vi "resonant.calculation vi_rrMD.vi"() -> ()   [LabVIEW 2012]
doc: "SciScan 1.2 160622"
uses:
  CommonResource VIs/Timing/Timer Commands.ctl
  Custom Controls/display palette control.ctl
  Custom Controls/scan mode main settings tab.ctl
  Custom Controls/pixel resolution resonant enum.ctl
  Custom Controls/MAIN Image panel reso tab Control type def.ctl
  Custom Controls/experiment type.ctl
  Custom Controls/advanced settings inner tab CTL.ctl
  Plugins/Macro Module/Macro Rule/subVIs/MacroRules_FGV_Commands.ctl
  Custom Controls/Histogram tab reso.ctl
  <vilib>/Utility/VariantDataType/Type.ctl
  GFG/GFGstringGet.vi
  GFG/GFGfpRefGet.vi
  GFG/GFGbooleanGet.vi
  GFG/GFGnumericGet.vi
  GFG/GFGDisplayRefsGet.vi
  GFG/GFGImageRefsGet.vi
  GFG/GFG library.lvlib
  <vilib>/Utility/VariantDataType/VariantType.lvlib
panel:
  out "Source VI 2":string
  out "ready for flystart?":bool
  out "Iteration":i32
  in  "String":string
  out "Source VI":string
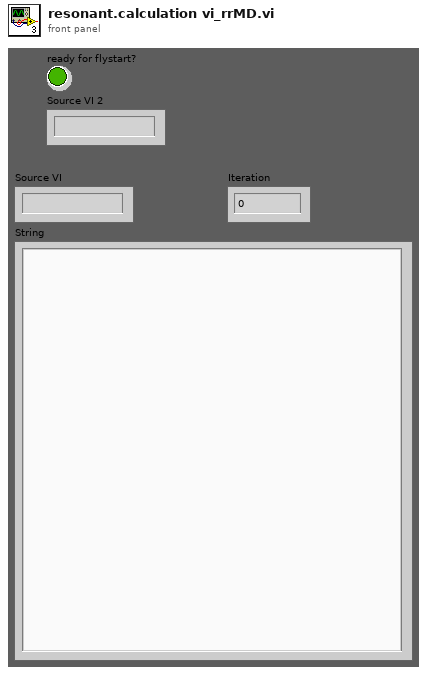
[diagram p1: front panel]
types:
  T1 = typedef "Timer Commands.ctl" = enum16{"Clear All", "Start", "Pause", "Check Time"}
  T2 = cluster{"WaveformChartRef":refnum<vi>, "DigitalRef":refnum<vi>, "ArrayRef":refnum<vi>, "TabControlRef":refnum<vi>, "EnumRef":refnum<vi>, "RingRef":refnum<vi>, "BooleanRef":refnum<vi>, "KnobRef":refnum<vi>, "SlideRef":refnum<vi>, "PathRef":refnum<vi>, "StringRef":refnum<vi>, "ComboBox":refnum<vi>, "WaveformGraphRef":refnum<vi>}
  T3 = typedef "display palette control.ctl" = enum16{"standard", "high clipping red", "low clipping blue", "high and low clipping", "high / low (full range)"}
  T4 = typedef "scan mode main settings tab.ctl" = enum32{"2D frame", "2D line scan", "general settings", "Z Stack", "piezo"}
  T5 = enum8{"Enabled", "Disabled", "Disabled and Grayed Out"}
  T6 = typedef "MAIN Image panel reso tab Control type def.ctl" = enum32{"Channel 1", "Channel 2", "Channel 3", "Channel 4", "Channel 5", "all channels", "RGB overlay", "ROI", "arbitrary line scan"}
  T7 = typedef "experiment type.ctl" = string
  T8 = enum32{"Page Enabled", "Page Disabled", "Page Disabled & Grayed"}
  T9 = typedef "advanced settings inner tab CTL.ctl" = enum32{"arb. frames", "AO", "AI", "channels", "trigger", "Zstack data"}
  T10 = typedef "MacroRules_FGV_Commands.ctl" = enum16{"Read File", "Get All", "Get Param and Flags"}
  T11 = typedef "Histogram tab reso.ctl" = enum32{"hist Ch 1", "hist Ch 4", "hist Ch 5", "hist Ch 3", "hist Ch 2"}
  T12 = cluster{"Channel 1 small":refnum<vi>, "Channel 2 small":refnum<vi>, "Channel 3 small":refnum<vi>, "Channel 4 small":refnum<vi>, "Channel 1 large":refnum<vi>, "Channel 2 large":refnum<vi>, "Channel 3 large":refnum<vi>, "Channel 4 large":refnum<vi>, "RGB overlay":refnum<vi>, "ROI Image display":refnum<vi>, "arb line scan display":refnum<vi>, "Channel 5 large":refnum<vi>}
  T13 = typedef "pixel resolution resonant enum.ctl" = enum16{"512 x  64", "512 x 128", "512 x 256", "512 x 512", "512 x arbitrary", "1024 x 512", "1024 x 1024", " 1024 x arbitrary", " 1536 x  512", " 1536 x arbitrary"}
  T14 = typedef "biotfile select.ctl" = enum16{"7962with5751_512px_40Mhz", "7962with5751_512px_50Mhz", "7961with5734_1024px_120Mhz or ext lasersync", "7962with5734_1024px_120Mhz or ext lasersync", "7962with5734_512px_120Mhz or ext lasersync", "7961with5734_512px_120Mhz or ext lasersync", "7962with5751_12kHz_512px_50MHz_4ch", "7962with5751_1536px_2ch_40Mhz", "7962with5751_1536px_2ch_50Mhz", "7962with5751_12kHz_1024px_2ch_50MHz"}
  T15 = typedef "LVStringsAndValuesArrayTypeDef.ctl" = cluster{"String":string, "Value":ext}[]
  T16 = typedef "IMAQ Image.ctl" = refnum<image>
  T17 = cluster{"Channel 1 small":T16, "Channel 2 small":T16, "Channel 3 small":T16, "Channel 4 small":T16, "Channel 1 large":T16, "Channel 2 large":T16, "Channel 3 large":T16, "Channel 4 large":T16, "RGB overlay":T16, "ROI Image display":T16, "arb line scan display":T16, "Channel 5 large":T16}
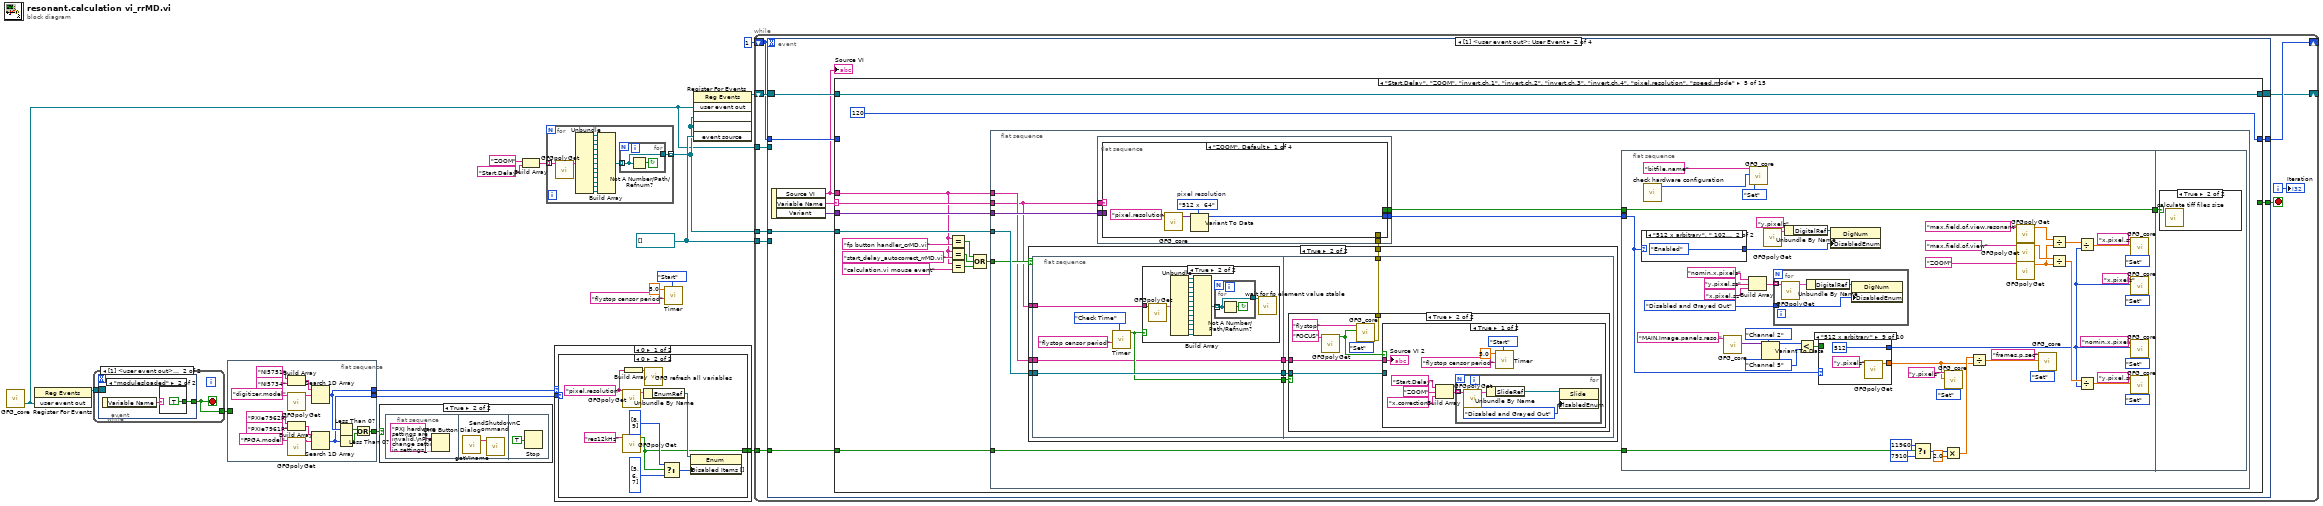
[diagram p0: block diagram]
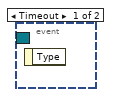
[diagram p3: hidden frame]
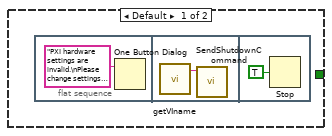
[diagram p5: hidden frame]
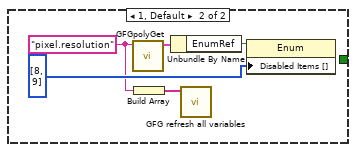
[diagram p6: hidden frame]
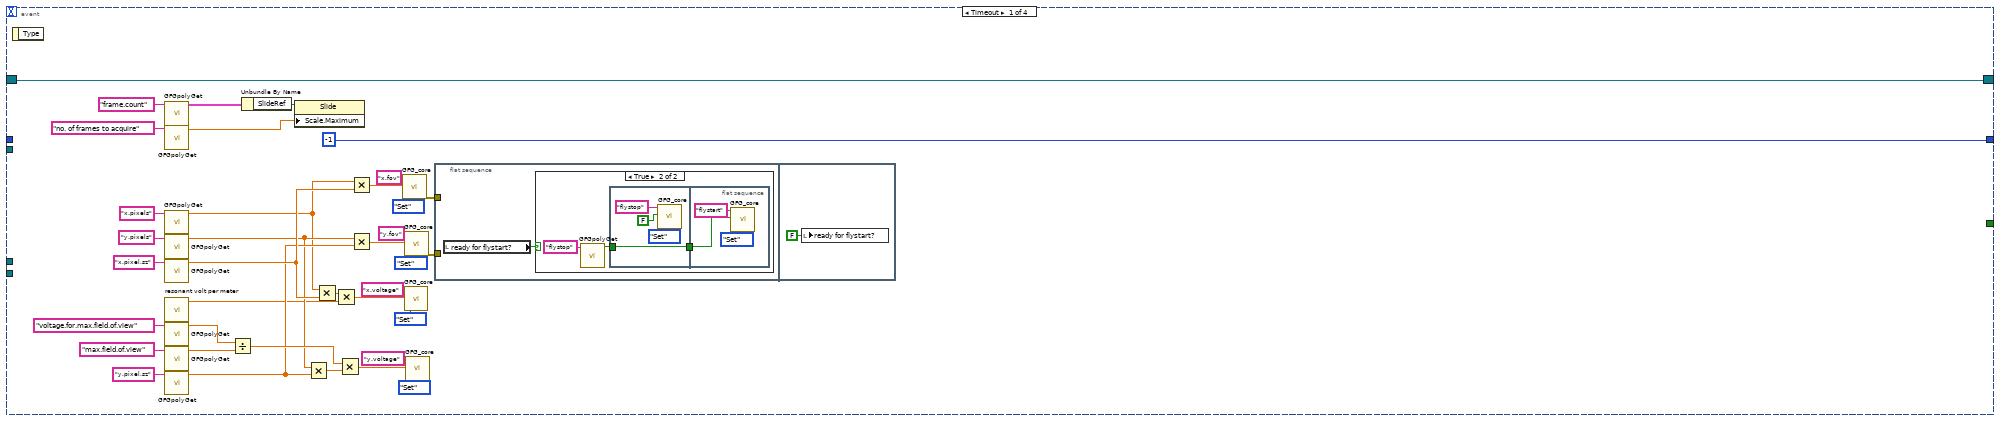
[diagram p7: hidden frame]
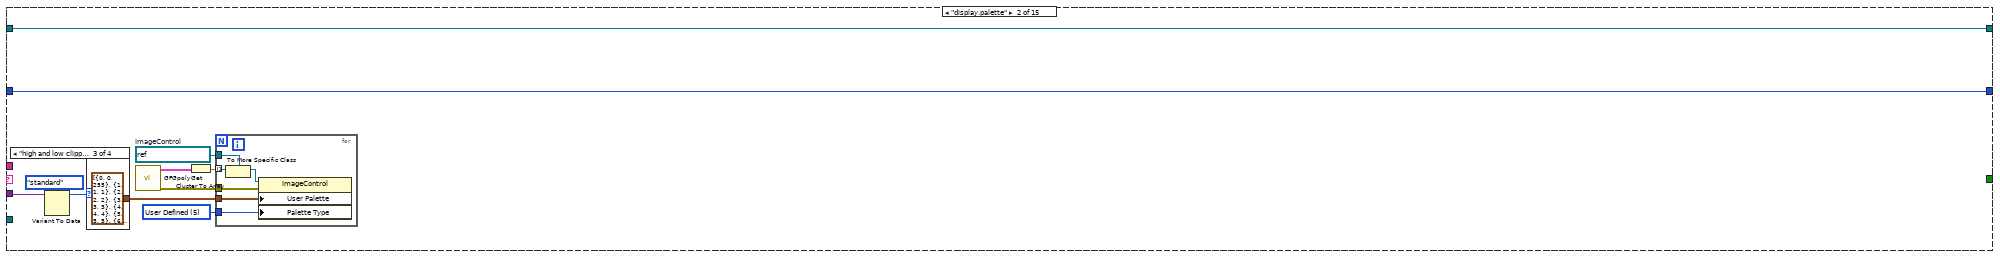
[diagram p10: hidden frame]
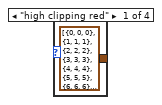
[diagram p11: hidden frame]
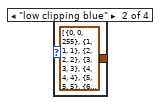
[diagram p12: hidden frame]
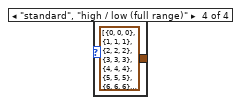
[diagram p13: hidden frame]
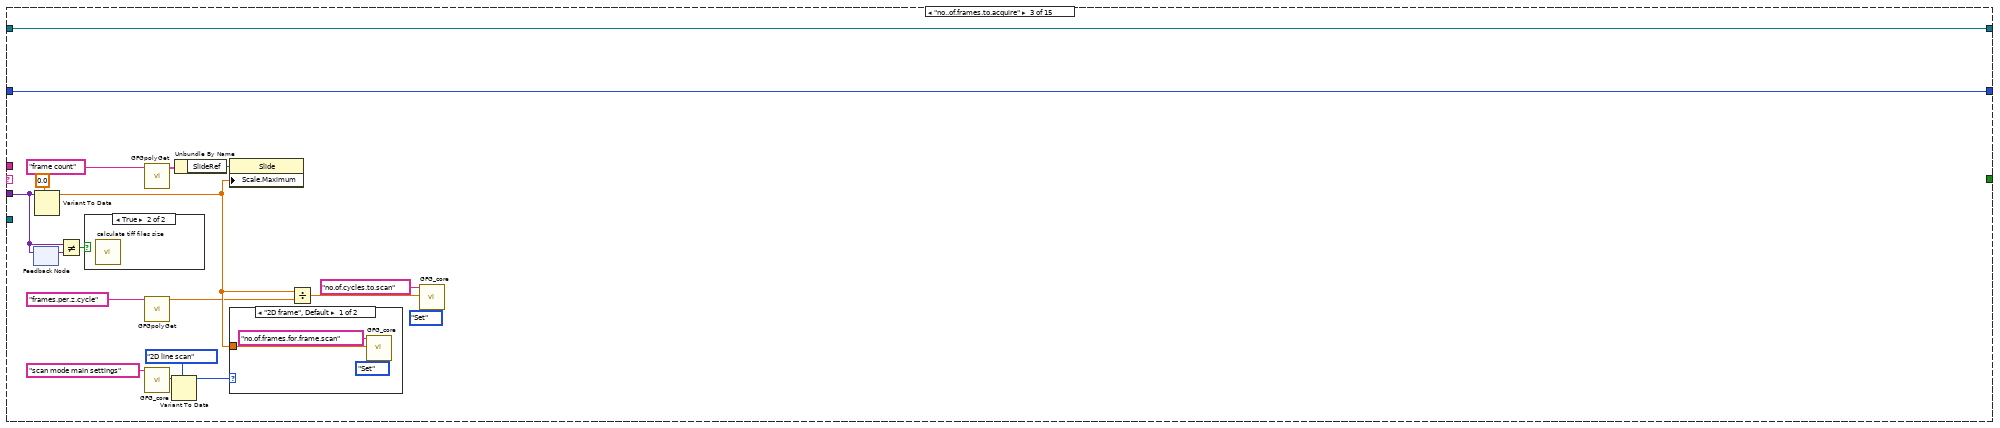
[diagram p14: hidden frame]
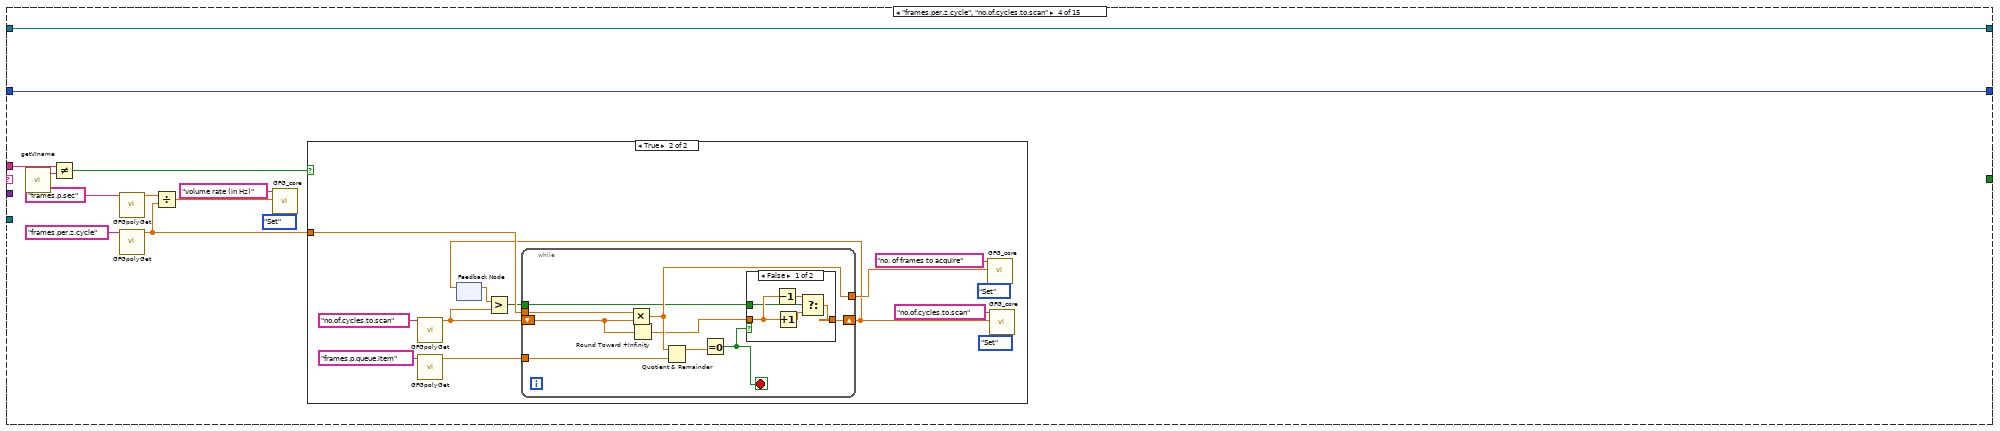
[diagram p17: hidden frame]
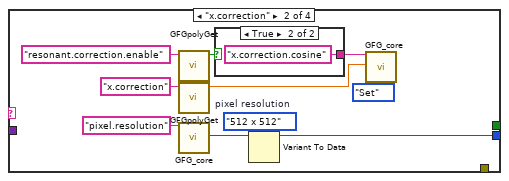
[diagram p20: hidden frame]
diagram:
  w11 = refnum<vi>[] [] ("event source")
  n1 = call "GFG_core.vi"() -> ("user event out"=w1:refnum<user-event>)  [unwired: 13 in, 6 out]
  n2 = register-events(w1) -> (reference out=w10:refnum<event-registration>)  [unwired: 2 in, 1 out]
  n3 = while {
    tunnel: w10 -> [w19]
    tunnel: [w18] -> w9
    stop <- w18 stop-if-true
    n4 = event shown="[1] <user event out>: User Event" {
      selector: w19 -> [_ _]
      dyn-events: _ -> [_ _]
      timeout: _ -> [_ _]
      tunnel: [_ w20] -> w18
      event Timeout {
        n5 = event-data() -> ()  [unwired: 1 in, 1 out]
      }
      event User Event {
        n6 = event-data() -> ("Variable Name"=w21:string)  [unwired: 1 in]
        n7 = case shown="\"modulesloaded\"" w21 {
          tunnel: [_ TRUE ("stop? (T)")] -> w20
          frame "False", Default {
          }
          frame "modulesloaded" {
          }
        }
      }
    }
  }
  n8 = flat-sequence {
    tunnel: [w25] -> w16
    tunnel: [w24] -> w15
    tunnel: [w23] -> w14
    tunnel: w9 -> [_]
    frame #0 {
      n9 = Build Array("NI5751", "NI5734") -> (w36:string[])
      n10 = call-poly "GFGpolyGet.vi"("Variable Name in"="digitizer.model") -> ("String"=w34:string)  [unwired: 9 in, 1 out]
      n11 = Build Array("PXIe7962R", "PXIe7961R") -> (w37:string[])
      n12 = call-poly "GFGpolyGet.vi"("Variable Name in"="FPGA.model") -> ("String"=w35:string)  [unwired: 9 in, 1 out]
      n13 = Search 1D Array(1D array=w36, element=w34) -> (index of element=w24:i32)  [unwired: 1 in]
      n14 = Search 1D Array(1D array=w37, element=w35) -> (index of element=w23:i32)  [unwired: 1 in]
      n15 = Less Than 0?(x=w24) -> (x < 0?=w27:bool)
      n16 = Less Than 0?(x=w23) -> (x < 0?=w26:bool)
      n17 = Or(x=w27, y=w26) -> (x .or. y?=w25:bool)
    }
  }
  n18 = case shown="True" w16 {
    frame False {
    }
    frame True {
      n19 = flat-sequence {
        frame #0 {
          n20 = One Button Dialog(message="PXI hardware settings are invalid.\nPlease change settings in settings_reso.ini\nSciScan will exit now. ") -> ()  [unwired: 1 in, 1 out]
        }
        frame #1 {
          n21 = call "getVIname.vi"() -> ("VI name"=w39:string)  [unwired: 19 in]
          n22 = call "SendShutdownCommand.vi"("Source VI"=w39) -> ()  [unwired: 11 in]
        }
        frame #2 {
          n23 = Stop(stop? (T)=TRUE) -> ()
        }
      }
    }
  }
  n24 = Build Array("ZOOM", "Start.Delay") -> (w6:string[])
  n25 = for {
    tunnel: w6 -> [w41] mode=indexing
    tunnel: [w42] -> w5 mode=indexing
    n26 = call-poly "GFGpolyGet.vi"("Variable Name in"=w41) -> ("output cluster"=w44:T2)  [unwired: 9 in, 1 out]
    n27 = Unbundle(w44) -> ("WaveformChartRef"=w55:refnum<vi>, "DigitalRef"=w54:refnum<vi>, "ArrayRef"=w53:refnum<vi>, "TabControlRef"=w52:refnum<vi>, "EnumRef"=w51:refnum<vi>, "RingRef"=w50:refnum<vi>, "BooleanRef"=w49:refnum<vi>, "KnobRef"=w48:refnum<vi>, "SlideRef"=w47:refnum<vi>, "PathRef"=w46:refnum<vi>, "StringRef"=w45:refnum<vi>, "ComboBox"=w56:refnum<vi>, "WaveformGraphRef"=w57:refnum<vi>)
    n28 = Build Array(w55, w54, w53, w52, w51, w50, w49, w48, w47, w46, w45, w56, w57) -> (w43:refnum<vi>[])
    n29 = for {
      tunnel: w43 -> [w58] mode=indexing
      tunnel: [w58] -> w42
      stop <- w59 continue-if-true
      n30 = Not A Number/Path/Refnum?(number/path/refnum=w58) -> (NaN/Path/Refnum?=w59:bool)
    }
  }
  n31 = case shown="0" w15 {
    tunnel: w14 -> [w61 _]
    tunnel: [w60 _] -> w13
    frame 0 {
      n32 = case shown="0" w61 {
        tunnel: [_ w66] -> w60
        frame Default {
          n33 = flat-sequence {
            frame #0 {
              n34 = One Button Dialog(message="PXI hardware settings are invalid.\nPlease change settings in settings_reso.ini\nSciScan will exit now. ") -> ()  [unwired: 1 in, 1 out]
            }
            frame #1 {
              n35 = call "getVIname.vi"() -> ("VI name"=w63:string)  [unwired: 19 in]
              n36 = call "SendShutdownCommand.vi"("Source VI"=w63) -> ()  [unwired: 11 in]
            }
            frame #2 {
              n37 = Stop(stop? (T)=TRUE) -> ()
            }
          }
        }
        frame 0 {
          w71 = "pixel.resolution" ("Variable Name in")
          n38 = call-poly "GFGpolyGet.vi"("Variable Name in"=w71) -> ("output cluster"=w72:T2)  [unwired: 9 in, 1 out]
          n39 = call-poly "GFGpolyGet.vi"("Variable Name in"="res12kHz") -> ("Boolean Value OUT"=w66:bool)  [unwired: 9 in, 1 out]
          n40 = Build Array(w71) -> (w65:string[])
          n41 = Unbundle By Name(w72) -> ("EnumRef"=w73:refnum<vi>)
          n42 = call "GFG refresh all variables.vi"("Variables to refresh"=w65) -> ()  [unwired: 11 in]
          n43 = Select(t=i32[] [8, 9] ("Disabled Items [] 2"), s=w66, f=i32[] [5, 6, 7] ("Disabled Items [] 2")) -> (s? t:f=w67:i32[])
          n44 = property class="Enum"(reference=w73, "Disabled Items []"=w67) -> ()  [unwired: 1 in, 2 out]
        }
      }
    }
    frame 1, Default {
      w74 = "pixel.resolution" ("Variable Name in")
      n45 = call-poly "GFGpolyGet.vi"("Variable Name in"=w74) -> ("output cluster"=w77:T2)  [unwired: 9 in, 1 out]
      n46 = Build Array(w74) -> (w75:string[])
      n47 = Unbundle By Name(w77) -> ("EnumRef"=w78:refnum<vi>)
      n48 = call "GFG refresh all variables.vi"("Variables to refresh"=w75) -> ()  [unwired: 11 in]
      n49 = property class="Enum"(reference=w78, "Disabled Items []"=i32[] [8, 9] ("Disabled Items [] 2")) -> ()  [unwired: 1 in, 2 out]
    }
  }
  n50 = call "Timer.vi"("Timer Command"=Timer_Commands."Start", "name qualifier (empty if unwired)"="flystop censor period", "Set Time IN (s)"=5.0) -> ()  [unwired: 3 in, 6 out]
  n51 = register-events(w1, w5, w5, w11) -> (reference out=w12:refnum<event-registration>)  [unwired: 2 in, 1 out]
  n52 = while {
    shift-right: [w86] -> _
    shift-left: 1 -> [w85]
    shift-right: [w82] -> _
    shift-left: w12 -> [w88]
    tunnel: w1 -> [w83]
    tunnel: w13 -> [w81]
    tunnel: w5 -> [w80]
    tunnel: w11 -> [w79]
    i -> [w84]
    stop <- w87 stop-if-true
    n53 = event shown="[1] <user event out>: User Event" {
      selector: w88 -> [w93 w143 w733 w750]
      dyn-events: [w93 w142 w731 w749] -> w82
      timeout: w85 -> [_ _ _ _]
      tunnel: [_ w146 _ _] -> w87
      tunnel: [-1 w145 -1 -1] -> w86
      tunnel: w85 -> [_ w144 _ _]
      tunnel: w83 -> [_ _ _ w743]
      tunnel: w81 -> [_ w141 _ _]
      tunnel: w80 -> [_ w140 w732 w747]
      tunnel: w79 -> [_ _ w730 w748]
      event Timeout {
        n54 = event-data() -> ()  [unwired: 1 in, 1 out]
        n55 = call-poly "GFGpolyGet.vi"("Variable Name in"="frame.count") -> ("output cluster"=w97:T2)  [unwired: 9 in, 1 out]
        n56 = call-poly "GFGpolyGet.vi"("Variable Name in"="no. of frames to acquire") -> ("Numeric"=w94:dbl)  [unwired: 8 in, 2 out]
        n57 = call-poly "GFGpolyGet.vi"("Variable Name in"="x.pixels") -> ("Numeric"=w89:dbl)  [unwired: 8 in, 2 out]
        n58 = call-poly "GFGpolyGet.vi"("Variable Name in"="y.pixels") -> ("Numeric"=w99:dbl)  [unwired: 8 in, 2 out]
        n59 = call-poly "GFGpolyGet.vi"("Variable Name in"="x.pixel.sz") -> ("Numeric"=w103:dbl)  [unwired: 8 in, 2 out]
        n60 = call "resonant volt per meter.vi"() -> ("volt/meter interpolated"=w92:dbl)  [unwired: 11 in]
        n61 = call-poly "GFGpolyGet.vi"("Variable Name in"="voltage.for.max.field.of.view") -> ("Numeric"=w111:dbl)  [unwired: 8 in, 2 out]
        n62 = call-poly "GFGpolyGet.vi"("Variable Name in"="max.field.of.view") -> ("Numeric"=w112:dbl)  [unwired: 8 in, 2 out]
        n63 = call-poly "GFGpolyGet.vi"("Variable Name in"="y.pixel.sz") -> ("Numeric"=w101:dbl)  [unwired: 8 in, 2 out]
        n64 = Divide(x=w111, y=w112) -> (x/y=w110:dbl)
        n65 = Unbundle By Name(w97) -> ("SlideRef"=w96:refnum<vi>)
        n66 = property class="Slide"(reference=w96, "Scale.Maximum"=w94) -> ()  [unwired: 1 in, 2 out]
        n67 = Multiply(x=w99, y=w101) -> (x*y=w100:dbl)
        n68 = Multiply(x=w89, y=w103) -> (x*y=w102:dbl)
        n69 = Multiply(x=w102, y=w92) -> (x*y=w105:dbl)
        n70 = Multiply(x=w110, y=w100) -> (x*y=w104:dbl)
        n71 = Multiply(x=w89, y=w103) -> (x*y=w120:dbl)
        n72 = Multiply(x=w99, y=w101) -> (x*y=w117:dbl)
        n73 = call "GFG_core.vi"("Variable Name in"="x.fov", "Variant in"=w120, "Action"=enum16{"Init", "Set", "Get"}."Set") -> ("error out"=w91:errorcluster)  [unwired: 10 in, 6 out]
        n74 = call "GFG_core.vi"("Variable Name in"="x.voltage", "Variant in"=w105, "Action"=enum16{"Init", "Set", "Get"}."Set") -> ()  [unwired: 10 in, 7 out]
        n75 = call "GFG_core.vi"("Variable Name in"="y.fov", "Variant in"=w117, "Action"=enum16{"Init", "Set", "Get"}."Set") -> ("error out"=w90:errorcluster)  [unwired: 10 in, 6 out]
        n76 = call "GFG_core.vi"("Variable Name in"="y.voltage", "Variant in"=w104, "Action"=enum16{"Init", "Set", "Get"}."Set") -> ()  [unwired: 10 in, 7 out]
        n77 = flat-sequence {
          tunnel: w91 -> [_]
          tunnel: w90 -> [_]
          frame #0 {
            n78 = local read "ready for flystart?"() -> (w126:bool)
            n79 = case shown="True" w126 {
              frame False {
              }
              frame True {
                n80 = call-poly "GFGpolyGet.vi"("Variable Name in"="flystop") -> ("Boolean Value OUT"=w128:bool)  [unwired: 9 in, 1 out]
                n81 = flat-sequence {
                  tunnel: w128 -> [w130]
                  tunnel: [w130] -> w127
                  tunnel: w127 -> [w134]
                  frame #0 {
                    n82 = call "GFG_core.vi"("Variable Name in"="flystop", "Variant in"=FALSE ("Boolean"), "Action"=enum16{"Init", "Set", "Get"}."Set") -> ()  [unwired: 10 in, 7 out]
                  }
                  frame #1 {
                    n83 = call "GFG_core.vi"("Variable Name in"="flystart", "Variant in"=w134, "Action"=enum16{"Init", "Set", "Get"}."Set") -> ()  [unwired: 10 in, 7 out]
                  }
                }
              }
            }
          }
          frame #1 {
            n84 = local write "ready for flystart?"(FALSE ("ready for flystart?")) -> ()
          }
        }
      }
      event User Event {
        n85 = event-data() -> ("Source VI"=w139:string, "Variable Name"=w147:string, "Variant"=w138:variant)  [unwired: 1 in]
        "Source VI" <- w139
        n86 = case shown="\"Start.Delay\", \"ZOOM\", \"invert.ch.1\", \"invert.ch.2\", \"invert.ch.3\", \"invert.ch.4\", \"pixel.resolution\", \"speed.mode\"" w147 {
          selector: w147 -> [_ _ _ _ w245 w441 w485 _ w521 _ w609 _ _ _ _]
          tunnel: [_ _ _ _ _ _ _ _ _ _ _ _ _ _ TRUE] -> w146
          tunnel: w138 -> [_ w160 w171 _ w244 w442 _ _ _ w564 _ w640 w693 w709 _]
          tunnel: [w149 w157 w185 w201 120 w440 w487 w515 w524 w560 150 w637 w685 w710 w725] -> w145
          tunnel: w144 -> [w149 w157 w185 w201 _ w440 w487 w515 w524 w561 _ w638 w685 w710 w725]
          tunnel: [w148 w150 w180 w200 w246 w439 w488 w514 w525 w559 w610 w633 w684 w703 w724] -> w142
          tunnel: w143 -> [w148 w150 w180 w200 w246 w439 w488 w514 w525 w559 w610 w633 w684 w703 w724]
          tunnel: w141 -> [_ _ _ _ w243 _ _ _ _ _ _ _ _ _ _]
          tunnel: w139 -> [_ _ _ w193 w234 _ _ _ _ _ _ _ _ _ _]
          tunnel: w140 -> [_ _ _ _ w241 _ _ _ _ _ _ _ _ _ _]
          frame Default {
          }
          frame "display.palette" {
            w152 = u32 5 items=["Grayscale", "Binary", "Gradient", "Rainbow", "Temperature", "User Defined"] ("Palette:Palette Type")
            w154 = refnum<vi> refnum  # ImageControl
            n87 = Variant To Data(type=display_palette_control."standard" ("display palette"), Variant=w160) -> (data=w158:T3)  [unwired: 1 in, 1 out]
            n88 = case shown="\"high and low clipping\"" w158 {
              tunnel: [cluster{"Red":u8, "Green":u8, "Blue":u8}[] [{"Red"=0, "Green"=0, "Blue"=0}, {"Red"=1, "Green"=1, "Blue"=1}, {"Red"=2, "Green"=2, "Blue"=2}, {"Red"=3, "Green"=3, "Blue"=3}, {"Red"=4, "Green"=4, "Blue"=4}, {"Red"=5, "Green"=5, "Blue"=5}, {"Red"=6, "Green"=6, "Blue"=6}, {"Red"=7, "Green"=7, "Blue"=7}, {"Red"=8, "Green"=8, "Blue"=8}, {"Red"=9, "Green"=9, "Blue"=9}, {"Red"=10, "Green"=10, "Blue"=10}, {"Red"=11, "Green"=11, "Blue"=11}, {"Red"=12, "Green"=12, "Blue"=12}, {"Red"=13, "Green"=13, "Blue"=13}, {"Red"=14, "Green"=14, "Blue"=14}, {"Red"=15, "Green"=15, "Blue"=15}, {"Red"=16, "Green"=16, "Blue"=16}, {"Red"=17, "Green"=17, "Blue"=17}, {"Red"=18, "Green"=18, "Blue"=18}, {"Red"=19, "Green"=19, "Blue"=19}, {"Red"=20, "Green"=20, "Blue"=20}, {"Red"=21, "Green"=21, "Blue"=21}, {"Red"=22, "Green"=22, "Blue"=22}, {"Red"=23, "Green"=23, "Blue"=23}, {"Red"=24, "Green"=24, "Blue"=24}, {"Red"=25, "Green"=25, "Blue"=25}, {"Red"=26, "Green"=26, "Blue"=26}, {"Red"=27, "Green"=27, "Blue"=27}, {"Red"=28, "Green"=28, "Blue"=28}, {"Red"=29, "Green"=29, "Blue"=29}, {"Red"=30, "Green"=30, "Blue"=30}, {"Red"=31, "Green"=31, "Blue"=31}, {"Red"=32, "Green"=32, "Blue"=32}, {"Red"=33, "Green"=33, "Blue"=33}, {"Red"=34, "Green"=34, "Blue"=34}, {"Red"=35, "Green"=35, "Blue"=35}, {"Red"=36, "Green"=36, "Blue"=36}, {"Red"=37, "Green"=37, "Blue"=37}, {"Red"=38, "Green"=38, "Blue"=38}, {"Red"=39, "Green"=39, "Blue"=39}, {"Red"=40, "Green"=40, "Blue"=40}, {"Red"=41, "Green"=41, "Blue"=41}, {"Red"=42, "Green"=42, "Blue"=42}, {"Red"=43, "Green"=43, "Blue"=43}, {"Red"=44, "Green"=44, "Blue"=44}, {"Red"=45, "Green"=45, "Blue"=45}, {"Red"=46, "Green"=46, "Blue"=46}, {"Red"=47, "Green"=47, "Blue"=47}, {"Red"=48, "Green"=48, "Blue"=48}, {"Red"=49, "Green"=49, "Blue"=49}, {"Red"=50, "Green"=50, "Blue"=50}, {"Red"=51, "Green"=51, "Blue"=51}, {"Red"=52, "Green"=52, "Blue"=52}, {"Red"=53, "Green"=53, "Blue"=53}, {"Red"=54, "Green"=54, "Blue"=54}, {"Red"=55, "Green"=55, "Blue"=55}, {"Red"=56, "Green"=56, "Blue"=56}, {"Red"=57, "Green"=57, "Blue"=57}, {"Red"=58, "Green"=58, "Blue"=58}, {"Red"=59, "Green"=59, "Blue"=59}, {"Red"=60, "Green"=60, "Blue"=60}, {"Red"=61, "Green"=61, "Blue"=61}, {"Red"=62, "Green"=62, "Blue"=62}, {"Red"=63, "Green"=63, "Blue"=63}, {"Red"=64, "Green"=64, "Blue"=64}, {"Red"=65, "Green"=65, "Blue"=65}, {"Red"=66, "Green"=66, "Blue"=66}, {"Red"=67, "Green"=67, "Blue"=67}, {"Red"=68, "Green"=68, "Blue"=68}, {"Red"=69, "Green"=69, "Blue"=69}, {"Red"=70, "Green"=70, "Blue"=70}, {"Red"=71, "Green"=71, "Blue"=71}, {"Red"=72, "Green"=72, "Blue"=72}, {"Red"=73, "Green"=73, "Blue"=73}, {"Red"=74, "Green"=74, "Blue"=74}, {"Red"=75, "Green"=75, "Blue"=75}, {"Red"=76, "Green"=76, "Blue"=76}, {"Red"=77, "Green"=77, "Blue"=77}, {"Red"=78, "Green"=78, "Blue"=78}, {"Red"=79, "Green"=79, "Blue"=79}, {"Red"=80, "Green"=80, "Blue"=80}, {"Red"=81, "Green"=81, "Blue"=81}, {"Red"=82, "Green"=82, "Blue"=82}, {"Red"=83, "Green"=83, "Blue"=83}, {"Red"=84, "Green"=84, "Blue"=84}, {"Red"=85, "Green"=85, "Blue"=85}, {"Red"=86, "Green"=86, "Blue"=86}, {"Red"=87, "Green"=87, "Blue"=87}, {"Red"=88, "Green"=88, "Blue"=88}, {"Red"=89, "Green"=89, "Blue"=89}, {"Red"=90, "Green"=90, "Blue"=90}, {"Red"=91, "Green"=91, "Blue"=91}, {"Red"=92, "Green"=92, "Blue"=92}, {"Red"=93, "Green"=93, "Blue"=93}, {"Red"=94, "Green"=94, "Blue"=94}, {"Red"=95, "Green"=95, "Blue"=95}, {"Red"=96, "Green"=96, "Blue"=96}, {"Red"=97, "Green"=97, "Blue"=97}, {"Red"=98, "Green"=98, "Blue"=98}, {"Red"=99, "Green"=99, "Blue"=99}, {"Red"=100, "Green"=100, "Blue"=100}, {"Red"=101, "Green"=101, "Blue"=101}, {"Red"=102, "Green"=102, "Blue"=102}, {"Red"=103, "Green"=103, "Blue"=103}, {"Red"=104, "Green"=104, "Blue"=104}, {"Red"=105, "Green"=105, "Blue"=105}, {"Red"=106, "Green"=106, "Blue"=106}, {"Red"=107, "Green"=107, "Blue"=107}, {"Red"=108, "Green"=108, "Blue"=108}, {"Red"=109, "Green"=109, "Blue"=109}, {"Red"=110, "Green"=110, "Blue"=110}, {"Red"=111, "Green"=111, "Blue"=111}, {"Red"=112, "Green"=112, "Blue"=112}, {"Red"=113, "Green"=113, "Blue"=113}, {"Red"=114, "Green"=114, "Blue"=114}, {"Red"=115, "Green"=115, "Blue"=115}, {"Red"=116, "Green"=116, "Blue"=116}, {"Red"=117, "Green"=117, "Blue"=117}, {"Red"=118, "Green"=118, "Blue"=118}, {"Red"=119, "Green"=119, "Blue"=119}, {"Red"=120, "Green"=120, "Blue"=120}, {"Red"=121, "Green"=121, "Blue"=121}, {"Red"=122, "Green"=122, "Blue"=122}, {"Red"=123, "Green"=123, "Blue"=123}, {"Red"=124, "Green"=124, "Blue"=124}, {"Red"=125, "Green"=125, "Blue"=125}, {"Red"=126, "Green"=126, "Blue"=126}, {"Red"=127, "Green"=127, "Blue"=127}, {"Red"=128, "Green"=128, "Blue"=128}, {"Red"=129, "Green"=129, "Blue"=129}, {"Red"=130, "Green"=130, "Blue"=130}, {"Red"=131, "Green"=131, "Blue"=131}, {"Red"=132, "Green"=132, "Blue"=132}, {"Red"=133, "Green"=133, "Blue"=133}, {"Red"=134, "Green"=134, "Blue"=134}, {"Red"=135, "Green"=135, "Blue"=135}, {"Red"=136, "Green"=136, "Blue"=136}, {"Red"=137, "Green"=137, "Blue"=137}, {"Red"=138, "Green"=138, "Blue"=138}, {"Red"=139, "Green"=139, "Blue"=139}, {"Red"=140, "Green"=140, "Blue"=140}, {"Red"=141, "Green"=141, "Blue"=141}, {"Red"=142, "Green"=142, "Blue"=142}, {"Red"=143, "Green"=143, "Blue"=143}, {"Red"=144, "Green"=144, "Blue"=144}, {"Red"=145, "Green"=145, "Blue"=145}, {"Red"=146, "Green"=146, "Blue"=146}, {"Red"=147, "Green"=147, "Blue"=147}, {"Red"=148, "Green"=148, "Blue"=148}, {"Red"=149, "Green"=149, "Blue"=149}, {"Red"=150, "Green"=150, "Blue"=150}, {"Red"=151, "Green"=151, "Blue"=151}, {"Red"=152, "Green"=152, "Blue"=152}, {"Red"=153, "Green"=153, "Blue"=153}, {"Red"=154, "Green"=154, "Blue"=154}, {"Red"=155, "Green"=155, "Blue"=155}, {"Red"=156, "Green"=156, "Blue"=156}, {"Red"=157, "Green"=157, "Blue"=157}, {"Red"=158, "Green"=158, "Blue"=158}, {"Red"=159, "Green"=159, "Blue"=159}, {"Red"=160, "Green"=160, "Blue"=160}, {"Red"=161, "Green"=161, "Blue"=161}, {"Red"=162, "Green"=162, "Blue"=162}, {"Red"=163, "Green"=163, "Blue"=163}, {"Red"=164, "Green"=164, "Blue"=164}, {"Red"=165, "Green"=165, "Blue"=165}, {"Red"=166, "Green"=166, "Blue"=166}, {"Red"=167, "Green"=167, "Blue"=167}, {"Red"=168, "Green"=168, "Blue"=168}, {"Red"=169, "Green"=169, "Blue"=169}, {"Red"=170, "Green"=170, "Blue"=170}, {"Red"=171, "Green"=171, "Blue"=171}, {"Red"=172, "Green"=172, "Blue"=172}, {"Red"=173, "Green"=173, "Blue"=173}, {"Red"=174, "Green"=174, "Blue"=174}, {"Red"=175, "Green"=175, "Blue"=175}, {"Red"=176, "Green"=176, "Blue"=176}, {"Red"=177, "Green"=177, "Blue"=177}, {"Red"=178, "Green"=178, "Blue"=178}, {"Red"=179, "Green"=179, "Blue"=179}, {"Red"=180, "Green"=180, "Blue"=180}, {"Red"=181, "Green"=181, "Blue"=181}, {"Red"=182, "Green"=182, "Blue"=182}, {"Red"=183, "Green"=183, "Blue"=183}, {"Red"=184, "Green"=184, "Blue"=184}, {"Red"=185, "Green"=185, "Blue"=185}, {"Red"=186, "Green"=186, "Blue"=186}, {"Red"=187, "Green"=187, "Blue"=187}, {"Red"=188, "Green"=188, "Blue"=188}, {"Red"=189, "Green"=189, "Blue"=189}, {"Red"=190, "Green"=190, "Blue"=190}, {"Red"=191, "Green"=191, "Blue"=191}, {"Red"=192, "Green"=192, "Blue"=192}, {"Red"=193, "Green"=193, "Blue"=193}, {"Red"=194, "Green"=194, "Blue"=194}, {"Red"=195, "Green"=195, "Blue"=195}, {"Red"=196, "Green"=196, "Blue"=196}, {"Red"=197, "Green"=197, "Blue"=197}, {"Red"=198, "Green"=198, "Blue"=198}, {"Red"=199, "Green"=199, "Blue"=199}, {"Red"=200, "Green"=200, "Blue"=200}, {"Red"=201, "Green"=201, "Blue"=201}, {"Red"=202, "Green"=202, "Blue"=202}, {"Red"=203, "Green"=203, "Blue"=203}, {"Red"=204, "Green"=204, "Blue"=204}, {"Red"=205, "Green"=205, "Blue"=205}, {"Red"=206, "Green"=206, "Blue"=206}, {"Red"=207, "Green"=207, "Blue"=207}, {"Red"=208, "Green"=208, "Blue"=208}, {"Red"=209, "Green"=209, "Blue"=209}, {"Red"=210, "Green"=210, "Blue"=210}, {"Red"=211, "Green"=211, "Blue"=211}, {"Red"=212, "Green"=212, "Blue"=212}, {"Red"=213, "Green"=213, "Blue"=213}, {"Red"=214, "Green"=214, "Blue"=214}, {"Red"=215, "Green"=215, "Blue"=215}, {"Red"=216, "Green"=216, "Blue"=216}, {"Red"=217, "Green"=217, "Blue"=217}, {"Red"=218, "Green"=218, "Blue"=218}, {"Red"=219, "Green"=219, "Blue"=219}, {"Red"=220, "Green"=220, "Blue"=220}, {"Red"=221, "Green"=221, "Blue"=221}, {"Red"=222, "Green"=222, "Blue"=222}, {"Red"=223, "Green"=223, "Blue"=223}, {"Red"=224, "Green"=224, "Blue"=224}, {"Red"=225, "Green"=225, "Blue"=225}, {"Red"=226, "Green"=226, "Blue"=226}, {"Red"=227, "Green"=227, "Blue"=227}, {"Red"=228, "Green"=228, "Blue"=228}, {"Red"=229, "Green"=229, "Blue"=229}, {"Red"=230, "Green"=230, "Blue"=230}, {"Red"=231, "Green"=231, "Blue"=231}, {"Red"=232, "Green"=232, "Blue"=232}, {"Red"=233, "Green"=233, "Blue"=233}, {"Red"=234, "Green"=234, "Blue"=234}, {"Red"=235, "Green"=235, "Blue"=235}, {"Red"=236, "Green"=236, "Blue"=236}, {"Red"=237, "Green"=237, "Blue"=237}, {"Red"=238, "Green"=238, "Blue"=238}, {"Red"=239, "Green"=239, "Blue"=239}, {"Red"=240, "Green"=240, "Blue"=240}, {"Red"=241, "Green"=241, "Blue"=241}, {"Red"=242, "Green"=242, "Blue"=242}, {"Red"=243, "Green"=243, "Blue"=243}, {"Red"=244, "Green"=244, "Blue"=244}, {"Red"=245, "Green"=245, "Blue"=245}, {"Red"=246, "Green"=246, "Blue"=246}, {"Red"=247, "Green"=247, "Blue"=247}, {"Red"=248, "Green"=248, "Blue"=248}, {"Red"=249, "Green"=249, "Blue"=249}, {"Red"=250, "Green"=250, "Blue"=250}, {"Red"=251, "Green"=251, "Blue"=251}, {"Red"=252, "Green"=252, "Blue"=252}, {"Red"=253, "Green"=253, "Blue"=253}, {"Red"=254, "Green"=254, "Blue"=254}, {"Red"=255, "Green"=0, "Blue"=0}] ("Color Palette") cluster{"Red":u8, "Green":u8, "Blue":u8}[] [{"Red"=0, "Green"=0, "Blue"=255}, {"Red"=1, "Green"=1, "Blue"=1}, {"Red"=2, "Green"=2, "Blue"=2}, {"Red"=3, "Green"=3, "Blue"=3}, {"Red"=4, "Green"=4, "Blue"=4}, {"Red"=5, "Green"=5, "Blue"=5}, {"Red"=6, "Green"=6, "Blue"=6}, {"Red"=7, "Green"=7, "Blue"=7}, {"Red"=8, "Green"=8, "Blue"=8}, {"Red"=9, "Green"=9, "Blue"=9}, {"Red"=10, "Green"=10, "Blue"=10}, {"Red"=11, "Green"=11, "Blue"=11}, {"Red"=12, "Green"=12, "Blue"=12}, {"Red"=13, "Green"=13, "Blue"=13}, {"Red"=14, "Green"=14, "Blue"=14}, {"Red"=15, "Green"=15, "Blue"=15}, {"Red"=16, "Green"=16, "Blue"=16}, {"Red"=17, "Green"=17, "Blue"=17}, {"Red"=18, "Green"=18, "Blue"=18}, {"Red"=19, "Green"=19, "Blue"=19}, {"Red"=20, "Green"=20, "Blue"=20}, {"Red"=21, "Green"=21, "Blue"=21}, {"Red"=22, "Green"=22, "Blue"=22}, {"Red"=23, "Green"=23, "Blue"=23}, {"Red"=24, "Green"=24, "Blue"=24}, {"Red"=25, "Green"=25, "Blue"=25}, {"Red"=26, "Green"=26, "Blue"=26}, {"Red"=27, "Green"=27, "Blue"=27}, {"Red"=28, "Green"=28, "Blue"=28}, {"Red"=29, "Green"=29, "Blue"=29}, {"Red"=30, "Green"=30, "Blue"=30}, {"Red"=31, "Green"=31, "Blue"=31}, {"Red"=32, "Green"=32, "Blue"=32}, {"Red"=33, "Green"=33, "Blue"=33}, {"Red"=34, "Green"=34, "Blue"=34}, {"Red"=35, "Green"=35, "Blue"=35}, {"Red"=36, "Green"=36, "Blue"=36}, {"Red"=37, "Green"=37, "Blue"=37}, {"Red"=38, "Green"=38, "Blue"=38}, {"Red"=39, "Green"=39, "Blue"=39}, {"Red"=40, "Green"=40, "Blue"=40}, {"Red"=41, "Green"=41, "Blue"=41}, {"Red"=42, "Green"=42, "Blue"=42}, {"Red"=43, "Green"=43, "Blue"=43}, {"Red"=44, "Green"=44, "Blue"=44}, {"Red"=45, "Green"=45, "Blue"=45}, {"Red"=46, "Green"=46, "Blue"=46}, {"Red"=47, "Green"=47, "Blue"=47}, {"Red"=48, "Green"=48, "Blue"=48}, {"Red"=49, "Green"=49, "Blue"=49}, {"Red"=50, "Green"=50, "Blue"=50}, {"Red"=51, "Green"=51, "Blue"=51}, {"Red"=52, "Green"=52, "Blue"=52}, {"Red"=53, "Green"=53, "Blue"=53}, {"Red"=54, "Green"=54, "Blue"=54}, {"Red"=55, "Green"=55, "Blue"=55}, {"Red"=56, "Green"=56, "Blue"=56}, {"Red"=57, "Green"=57, "Blue"=57}, {"Red"=58, "Green"=58, "Blue"=58}, {"Red"=59, "Green"=59, "Blue"=59}, {"Red"=60, "Green"=60, "Blue"=60}, {"Red"=61, "Green"=61, "Blue"=61}, {"Red"=62, "Green"=62, "Blue"=62}, {"Red"=63, "Green"=63, "Blue"=63}, {"Red"=64, "Green"=64, "Blue"=64}, {"Red"=65, "Green"=65, "Blue"=65}, {"Red"=66, "Green"=66, "Blue"=66}, {"Red"=67, "Green"=67, "Blue"=67}, {"Red"=68, "Green"=68, "Blue"=68}, {"Red"=69, "Green"=69, "Blue"=69}, {"Red"=70, "Green"=70, "Blue"=70}, {"Red"=71, "Green"=71, "Blue"=71}, {"Red"=72, "Green"=72, "Blue"=72}, {"Red"=73, "Green"=73, "Blue"=73}, {"Red"=74, "Green"=74, "Blue"=74}, {"Red"=75, "Green"=75, "Blue"=75}, {"Red"=76, "Green"=76, "Blue"=76}, {"Red"=77, "Green"=77, "Blue"=77}, {"Red"=78, "Green"=78, "Blue"=78}, {"Red"=79, "Green"=79, "Blue"=79}, {"Red"=80, "Green"=80, "Blue"=80}, {"Red"=81, "Green"=81, "Blue"=81}, {"Red"=82, "Green"=82, "Blue"=82}, {"Red"=83, "Green"=83, "Blue"=83}, {"Red"=84, "Green"=84, "Blue"=84}, {"Red"=85, "Green"=85, "Blue"=85}, {"Red"=86, "Green"=86, "Blue"=86}, {"Red"=87, "Green"=87, "Blue"=87}, {"Red"=88, "Green"=88, "Blue"=88}, {"Red"=89, "Green"=89, "Blue"=89}, {"Red"=90, "Green"=90, "Blue"=90}, {"Red"=91, "Green"=91, "Blue"=91}, {"Red"=92, "Green"=92, "Blue"=92}, {"Red"=93, "Green"=93, "Blue"=93}, {"Red"=94, "Green"=94, "Blue"=94}, {"Red"=95, "Green"=95, "Blue"=95}, {"Red"=96, "Green"=96, "Blue"=96}, {"Red"=97, "Green"=97, "Blue"=97}, {"Red"=98, "Green"=98, "Blue"=98}, {"Red"=99, "Green"=99, "Blue"=99}, {"Red"=100, "Green"=100, "Blue"=100}, {"Red"=101, "Green"=101, "Blue"=101}, {"Red"=102, "Green"=102, "Blue"=102}, {"Red"=103, "Green"=103, "Blue"=103}, {"Red"=104, "Green"=104, "Blue"=104}, {"Red"=105, "Green"=105, "Blue"=105}, {"Red"=106, "Green"=106, "Blue"=106}, {"Red"=107, "Green"=107, "Blue"=107}, {"Red"=108, "Green"=108, "Blue"=108}, {"Red"=109, "Green"=109, "Blue"=109}, {"Red"=110, "Green"=110, "Blue"=110}, {"Red"=111, "Green"=111, "Blue"=111}, {"Red"=112, "Green"=112, "Blue"=112}, {"Red"=113, "Green"=113, "Blue"=113}, {"Red"=114, "Green"=114, "Blue"=114}, {"Red"=115, "Green"=115, "Blue"=115}, {"Red"=116, "Green"=116, "Blue"=116}, {"Red"=117, "Green"=117, "Blue"=117}, {"Red"=118, "Green"=118, "Blue"=118}, {"Red"=119, "Green"=119, "Blue"=119}, {"Red"=120, "Green"=120, "Blue"=120}, {"Red"=121, "Green"=121, "Blue"=121}, {"Red"=122, "Green"=122, "Blue"=122}, {"Red"=123, "Green"=123, "Blue"=123}, {"Red"=124, "Green"=124, "Blue"=124}, {"Red"=125, "Green"=125, "Blue"=125}, {"Red"=126, "Green"=126, "Blue"=126}, {"Red"=127, "Green"=127, "Blue"=127}, {"Red"=128, "Green"=128, "Blue"=128}, {"Red"=129, "Green"=129, "Blue"=129}, {"Red"=130, "Green"=130, "Blue"=130}, {"Red"=131, "Green"=131, "Blue"=131}, {"Red"=132, "Green"=132, "Blue"=132}, {"Red"=133, "Green"=133, "Blue"=133}, {"Red"=134, "Green"=134, "Blue"=134}, {"Red"=135, "Green"=135, "Blue"=135}, {"Red"=136, "Green"=136, "Blue"=136}, {"Red"=137, "Green"=137, "Blue"=137}, {"Red"=138, "Green"=138, "Blue"=138}, {"Red"=139, "Green"=139, "Blue"=139}, {"Red"=140, "Green"=140, "Blue"=140}, {"Red"=141, "Green"=141, "Blue"=141}, {"Red"=142, "Green"=142, "Blue"=142}, {"Red"=143, "Green"=143, "Blue"=143}, {"Red"=144, "Green"=144, "Blue"=144}, {"Red"=145, "Green"=145, "Blue"=145}, {"Red"=146, "Green"=146, "Blue"=146}, {"Red"=147, "Green"=147, "Blue"=147}, {"Red"=148, "Green"=148, "Blue"=148}, {"Red"=149, "Green"=149, "Blue"=149}, {"Red"=150, "Green"=150, "Blue"=150}, {"Red"=151, "Green"=151, "Blue"=151}, {"Red"=152, "Green"=152, "Blue"=152}, {"Red"=153, "Green"=153, "Blue"=153}, {"Red"=154, "Green"=154, "Blue"=154}, {"Red"=155, "Green"=155, "Blue"=155}, {"Red"=156, "Green"=156, "Blue"=156}, {"Red"=157, "Green"=157, "Blue"=157}, {"Red"=158, "Green"=158, "Blue"=158}, {"Red"=159, "Green"=159, "Blue"=159}, {"Red"=160, "Green"=160, "Blue"=160}, {"Red"=161, "Green"=161, "Blue"=161}, {"Red"=162, "Green"=162, "Blue"=162}, {"Red"=163, "Green"=163, "Blue"=163}, {"Red"=164, "Green"=164, "Blue"=164}, {"Red"=165, "Green"=165, "Blue"=165}, {"Red"=166, "Green"=166, "Blue"=166}, {"Red"=167, "Green"=167, "Blue"=167}, {"Red"=168, "Green"=168, "Blue"=168}, {"Red"=169, "Green"=169, "Blue"=169}, {"Red"=170, "Green"=170, "Blue"=170}, {"Red"=171, "Green"=171, "Blue"=171}, {"Red"=172, "Green"=172, "Blue"=172}, {"Red"=173, "Green"=173, "Blue"=173}, {"Red"=174, "Green"=174, "Blue"=174}, {"Red"=175, "Green"=175, "Blue"=175}, {"Red"=176, "Green"=176, "Blue"=176}, {"Red"=177, "Green"=177, "Blue"=177}, {"Red"=178, "Green"=178, "Blue"=178}, {"Red"=179, "Green"=179, "Blue"=179}, {"Red"=180, "Green"=180, "Blue"=180}, {"Red"=181, "Green"=181, "Blue"=181}, {"Red"=182, "Green"=182, "Blue"=182}, {"Red"=183, "Green"=183, "Blue"=183}, {"Red"=184, "Green"=184, "Blue"=184}, {"Red"=185, "Green"=185, "Blue"=185}, {"Red"=186, "Green"=186, "Blue"=186}, {"Red"=187, "Green"=187, "Blue"=187}, {"Red"=188, "Green"=188, "Blue"=188}, {"Red"=189, "Green"=189, "Blue"=189}, {"Red"=190, "Green"=190, "Blue"=190}, {"Red"=191, "Green"=191, "Blue"=191}, {"Red"=192, "Green"=192, "Blue"=192}, {"Red"=193, "Green"=193, "Blue"=193}, {"Red"=194, "Green"=194, "Blue"=194}, {"Red"=195, "Green"=195, "Blue"=195}, {"Red"=196, "Green"=196, "Blue"=196}, {"Red"=197, "Green"=197, "Blue"=197}, {"Red"=198, "Green"=198, "Blue"=198}, {"Red"=199, "Green"=199, "Blue"=199}, {"Red"=200, "Green"=200, "Blue"=200}, {"Red"=201, "Green"=201, "Blue"=201}, {"Red"=202, "Green"=202, "Blue"=202}, {"Red"=203, "Green"=203, "Blue"=203}, {"Red"=204, "Green"=204, "Blue"=204}, {"Red"=205, "Green"=205, "Blue"=205}, {"Red"=206, "Green"=206, "Blue"=206}, {"Red"=207, "Green"=207, "Blue"=207}, {"Red"=208, "Green"=208, "Blue"=208}, {"Red"=209, "Green"=209, "Blue"=209}, {"Red"=210, "Green"=210, "Blue"=210}, {"Red"=211, "Green"=211, "Blue"=211}, {"Red"=212, "Green"=212, "Blue"=212}, {"Red"=213, "Green"=213, "Blue"=213}, {"Red"=214, "Green"=214, "Blue"=214}, {"Red"=215, "Green"=215, "Blue"=215}, {"Red"=216, "Green"=216, "Blue"=216}, {"Red"=217, "Green"=217, "Blue"=217}, {"Red"=218, "Green"=218, "Blue"=218}, {"Red"=219, "Green"=219, "Blue"=219}, {"Red"=220, "Green"=220, "Blue"=220}, {"Red"=221, "Green"=221, "Blue"=221}, {"Red"=222, "Green"=222, "Blue"=222}, {"Red"=223, "Green"=223, "Blue"=223}, {"Red"=224, "Green"=224, "Blue"=224}, {"Red"=225, "Green"=225, "Blue"=225}, {"Red"=226, "Green"=226, "Blue"=226}, {"Red"=227, "Green"=227, "Blue"=227}, {"Red"=228, "Green"=228, "Blue"=228}, {"Red"=229, "Green"=229, "Blue"=229}, {"Red"=230, "Green"=230, "Blue"=230}, {"Red"=231, "Green"=231, "Blue"=231}, {"Red"=232, "Green"=232, "Blue"=232}, {"Red"=233, "Green"=233, "Blue"=233}, {"Red"=234, "Green"=234, "Blue"=234}, {"Red"=235, "Green"=235, "Blue"=235}, {"Red"=236, "Green"=236, "Blue"=236}, {"Red"=237, "Green"=237, "Blue"=237}, {"Red"=238, "Green"=238, "Blue"=238}, {"Red"=239, "Green"=239, "Blue"=239}, {"Red"=240, "Green"=240, "Blue"=240}, {"Red"=241, "Green"=241, "Blue"=241}, {"Red"=242, "Green"=242, "Blue"=242}, {"Red"=243, "Green"=243, "Blue"=243}, {"Red"=244, "Green"=244, "Blue"=244}, {"Red"=245, "Green"=245, "Blue"=245}, {"Red"=246, "Green"=246, "Blue"=246}, {"Red"=247, "Green"=247, "Blue"=247}, {"Red"=248, "Green"=248, "Blue"=248}, {"Red"=249, "Green"=249, "Blue"=249}, {"Red"=250, "Green"=250, "Blue"=250}, {"Red"=251, "Green"=251, "Blue"=251}, {"Red"=252, "Green"=252, "Blue"=252}, {"Red"=253, "Green"=253, "Blue"=253}, {"Red"=254, "Green"=254, "Blue"=254}, {"Red"=255, "Green"=255, "Blue"=255}] ("Color Palette") cluster{"Red":u8, "Green":u8, "Blue":u8}[] [{"Red"=0, "Green"=0, "Blue"=255}, {"Red"=1, "Green"=1, "Blue"=1}, {"Red"=2, "Green"=2, "Blue"=2}, {"Red"=3, "Green"=3, "Blue"=3}, {"Red"=4, "Green"=4, "Blue"=4}, {"Red"=5, "Green"=5, "Blue"=5}, {"Red"=6, "Green"=6, "Blue"=6}, {"Red"=7, "Green"=7, "Blue"=7}, {"Red"=8, "Green"=8, "Blue"=8}, {"Red"=9, "Green"=9, "Blue"=9}, {"Red"=10, "Green"=10, "Blue"=10}, {"Red"=11, "Green"=11, "Blue"=11}, {"Red"=12, "Green"=12, "Blue"=12}, {"Red"=13, "Green"=13, "Blue"=13}, {"Red"=14, "Green"=14, "Blue"=14}, {"Red"=15, "Green"=15, "Blue"=15}, {"Red"=16, "Green"=16, "Blue"=16}, {"Red"=17, "Green"=17, "Blue"=17}, {"Red"=18, "Green"=18, "Blue"=18}, {"Red"=19, "Green"=19, "Blue"=19}, {"Red"=20, "Green"=20, "Blue"=20}, {"Red"=21, "Green"=21, "Blue"=21}, {"Red"=22, "Green"=22, "Blue"=22}, {"Red"=23, "Green"=23, "Blue"=23}, {"Red"=24, "Green"=24, "Blue"=24}, {"Red"=25, "Green"=25, "Blue"=25}, {"Red"=26, "Green"=26, "Blue"=26}, {"Red"=27, "Green"=27, "Blue"=27}, {"Red"=28, "Green"=28, "Blue"=28}, {"Red"=29, "Green"=29, "Blue"=29}, {"Red"=30, "Green"=30, "Blue"=30}, {"Red"=31, "Green"=31, "Blue"=31}, {"Red"=32, "Green"=32, "Blue"=32}, {"Red"=33, "Green"=33, "Blue"=33}, {"Red"=34, "Green"=34, "Blue"=34}, {"Red"=35, "Green"=35, "Blue"=35}, {"Red"=36, "Green"=36, "Blue"=36}, {"Red"=37, "Green"=37, "Blue"=37}, {"Red"=38, "Green"=38, "Blue"=38}, {"Red"=39, "Green"=39, "Blue"=39}, {"Red"=40, "Green"=40, "Blue"=40}, {"Red"=41, "Green"=41, "Blue"=41}, {"Red"=42, "Green"=42, "Blue"=42}, {"Red"=43, "Green"=43, "Blue"=43}, {"Red"=44, "Green"=44, "Blue"=44}, {"Red"=45, "Green"=45, "Blue"=45}, {"Red"=46, "Green"=46, "Blue"=46}, {"Red"=47, "Green"=47, "Blue"=47}, {"Red"=48, "Green"=48, "Blue"=48}, {"Red"=49, "Green"=49, "Blue"=49}, {"Red"=50, "Green"=50, "Blue"=50}, {"Red"=51, "Green"=51, "Blue"=51}, {"Red"=52, "Green"=52, "Blue"=52}, {"Red"=53, "Green"=53, "Blue"=53}, {"Red"=54, "Green"=54, "Blue"=54}, {"Red"=55, "Green"=55, "Blue"=55}, {"Red"=56, "Green"=56, "Blue"=56}, {"Red"=57, "Green"=57, "Blue"=57}, {"Red"=58, "Green"=58, "Blue"=58}, {"Red"=59, "Green"=59, "Blue"=59}, {"Red"=60, "Green"=60, "Blue"=60}, {"Red"=61, "Green"=61, "Blue"=61}, {"Red"=62, "Green"=62, "Blue"=62}, {"Red"=63, "Green"=63, "Blue"=63}, {"Red"=64, "Green"=64, "Blue"=64}, {"Red"=65, "Green"=65, "Blue"=65}, {"Red"=66, "Green"=66, "Blue"=66}, {"Red"=67, "Green"=67, "Blue"=67}, {"Red"=68, "Green"=68, "Blue"=68}, {"Red"=69, "Green"=69, "Blue"=69}, {"Red"=70, "Green"=70, "Blue"=70}, {"Red"=71, "Green"=71, "Blue"=71}, {"Red"=72, "Green"=72, "Blue"=72}, {"Red"=73, "Green"=73, "Blue"=73}, {"Red"=74, "Green"=74, "Blue"=74}, {"Red"=75, "Green"=75, "Blue"=75}, {"Red"=76, "Green"=76, "Blue"=76}, {"Red"=77, "Green"=77, "Blue"=77}, {"Red"=78, "Green"=78, "Blue"=78}, {"Red"=79, "Green"=79, "Blue"=79}, {"Red"=80, "Green"=80, "Blue"=80}, {"Red"=81, "Green"=81, "Blue"=81}, {"Red"=82, "Green"=82, "Blue"=82}, {"Red"=83, "Green"=83, "Blue"=83}, {"Red"=84, "Green"=84, "Blue"=84}, {"Red"=85, "Green"=85, "Blue"=85}, {"Red"=86, "Green"=86, "Blue"=86}, {"Red"=87, "Green"=87, "Blue"=87}, {"Red"=88, "Green"=88, "Blue"=88}, {"Red"=89, "Green"=89, "Blue"=89}, {"Red"=90, "Green"=90, "Blue"=90}, {"Red"=91, "Green"=91, "Blue"=91}, {"Red"=92, "Green"=92, "Blue"=92}, {"Red"=93, "Green"=93, "Blue"=93}, {"Red"=94, "Green"=94, "Blue"=94}, {"Red"=95, "Green"=95, "Blue"=95}, {"Red"=96, "Green"=96, "Blue"=96}, {"Red"=97, "Green"=97, "Blue"=97}, {"Red"=98, "Green"=98, "Blue"=98}, {"Red"=99, "Green"=99, "Blue"=99}, {"Red"=100, "Green"=100, "Blue"=100}, {"Red"=101, "Green"=101, "Blue"=101}, {"Red"=102, "Green"=102, "Blue"=102}, {"Red"=103, "Green"=103, "Blue"=103}, {"Red"=104, "Green"=104, "Blue"=104}, {"Red"=105, "Green"=105, "Blue"=105}, {"Red"=106, "Green"=106, "Blue"=106}, {"Red"=107, "Green"=107, "Blue"=107}, {"Red"=108, "Green"=108, "Blue"=108}, {"Red"=109, "Green"=109, "Blue"=109}, {"Red"=110, "Green"=110, "Blue"=110}, {"Red"=111, "Green"=111, "Blue"=111}, {"Red"=112, "Green"=112, "Blue"=112}, {"Red"=113, "Green"=113, "Blue"=113}, {"Red"=114, "Green"=114, "Blue"=114}, {"Red"=115, "Green"=115, "Blue"=115}, {"Red"=116, "Green"=116, "Blue"=116}, {"Red"=117, "Green"=117, "Blue"=117}, {"Red"=118, "Green"=118, "Blue"=118}, {"Red"=119, "Green"=119, "Blue"=119}, {"Red"=120, "Green"=120, "Blue"=120}, {"Red"=121, "Green"=121, "Blue"=121}, {"Red"=122, "Green"=122, "Blue"=122}, {"Red"=123, "Green"=123, "Blue"=123}, {"Red"=124, "Green"=124, "Blue"=124}, {"Red"=125, "Green"=125, "Blue"=125}, {"Red"=126, "Green"=126, "Blue"=126}, {"Red"=127, "Green"=127, "Blue"=127}, {"Red"=128, "Green"=128, "Blue"=128}, {"Red"=129, "Green"=129, "Blue"=129}, {"Red"=130, "Green"=130, "Blue"=130}, {"Red"=131, "Green"=131, "Blue"=131}, {"Red"=132, "Green"=132, "Blue"=132}, {"Red"=133, "Green"=133, "Blue"=133}, {"Red"=134, "Green"=134, "Blue"=134}, {"Red"=135, "Green"=135, "Blue"=135}, {"Red"=136, "Green"=136, "Blue"=136}, {"Red"=137, "Green"=137, "Blue"=137}, {"Red"=138, "Green"=138, "Blue"=138}, {"Red"=139, "Green"=139, "Blue"=139}, {"Red"=140, "Green"=140, "Blue"=140}, {"Red"=141, "Green"=141, "Blue"=141}, {"Red"=142, "Green"=142, "Blue"=142}, {"Red"=143, "Green"=143, "Blue"=143}, {"Red"=144, "Green"=144, "Blue"=144}, {"Red"=145, "Green"=145, "Blue"=145}, {"Red"=146, "Green"=146, "Blue"=146}, {"Red"=147, "Green"=147, "Blue"=147}, {"Red"=148, "Green"=148, "Blue"=148}, {"Red"=149, "Green"=149, "Blue"=149}, {"Red"=150, "Green"=150, "Blue"=150}, {"Red"=151, "Green"=151, "Blue"=151}, {"Red"=152, "Green"=152, "Blue"=152}, {"Red"=153, "Green"=153, "Blue"=153}, {"Red"=154, "Green"=154, "Blue"=154}, {"Red"=155, "Green"=155, "Blue"=155}, {"Red"=156, "Green"=156, "Blue"=156}, {"Red"=157, "Green"=157, "Blue"=157}, {"Red"=158, "Green"=158, "Blue"=158}, {"Red"=159, "Green"=159, "Blue"=159}, {"Red"=160, "Green"=160, "Blue"=160}, {"Red"=161, "Green"=161, "Blue"=161}, {"Red"=162, "Green"=162, "Blue"=162}, {"Red"=163, "Green"=163, "Blue"=163}, {"Red"=164, "Green"=164, "Blue"=164}, {"Red"=165, "Green"=165, "Blue"=165}, {"Red"=166, "Green"=166, "Blue"=166}, {"Red"=167, "Green"=167, "Blue"=167}, {"Red"=168, "Green"=168, "Blue"=168}, {"Red"=169, "Green"=169, "Blue"=169}, {"Red"=170, "Green"=170, "Blue"=170}, {"Red"=171, "Green"=171, "Blue"=171}, {"Red"=172, "Green"=172, "Blue"=172}, {"Red"=173, "Green"=173, "Blue"=173}, {"Red"=174, "Green"=174, "Blue"=174}, {"Red"=175, "Green"=175, "Blue"=175}, {"Red"=176, "Green"=176, "Blue"=176}, {"Red"=177, "Green"=177, "Blue"=177}, {"Red"=178, "Green"=178, "Blue"=178}, {"Red"=179, "Green"=179, "Blue"=179}, {"Red"=180, "Green"=180, "Blue"=180}, {"Red"=181, "Green"=181, "Blue"=181}, {"Red"=182, "Green"=182, "Blue"=182}, {"Red"=183, "Green"=183, "Blue"=183}, {"Red"=184, "Green"=184, "Blue"=184}, {"Red"=185, "Green"=185, "Blue"=185}, {"Red"=186, "Green"=186, "Blue"=186}, {"Red"=187, "Green"=187, "Blue"=187}, {"Red"=188, "Green"=188, "Blue"=188}, {"Red"=189, "Green"=189, "Blue"=189}, {"Red"=190, "Green"=190, "Blue"=190}, {"Red"=191, "Green"=191, "Blue"=191}, {"Red"=192, "Green"=192, "Blue"=192}, {"Red"=193, "Green"=193, "Blue"=193}, {"Red"=194, "Green"=194, "Blue"=194}, {"Red"=195, "Green"=195, "Blue"=195}, {"Red"=196, "Green"=196, "Blue"=196}, {"Red"=197, "Green"=197, "Blue"=197}, {"Red"=198, "Green"=198, "Blue"=198}, {"Red"=199, "Green"=199, "Blue"=199}, {"Red"=200, "Green"=200, "Blue"=200}, {"Red"=201, "Green"=201, "Blue"=201}, {"Red"=202, "Green"=202, "Blue"=202}, {"Red"=203, "Green"=203, "Blue"=203}, {"Red"=204, "Green"=204, "Blue"=204}, {"Red"=205, "Green"=205, "Blue"=205}, {"Red"=206, "Green"=206, "Blue"=206}, {"Red"=207, "Green"=207, "Blue"=207}, {"Red"=208, "Green"=208, "Blue"=208}, {"Red"=209, "Green"=209, "Blue"=209}, {"Red"=210, "Green"=210, "Blue"=210}, {"Red"=211, "Green"=211, "Blue"=211}, {"Red"=212, "Green"=212, "Blue"=212}, {"Red"=213, "Green"=213, "Blue"=213}, {"Red"=214, "Green"=214, "Blue"=214}, {"Red"=215, "Green"=215, "Blue"=215}, {"Red"=216, "Green"=216, "Blue"=216}, {"Red"=217, "Green"=217, "Blue"=217}, {"Red"=218, "Green"=218, "Blue"=218}, {"Red"=219, "Green"=219, "Blue"=219}, {"Red"=220, "Green"=220, "Blue"=220}, {"Red"=221, "Green"=221, "Blue"=221}, {"Red"=222, "Green"=222, "Blue"=222}, {"Red"=223, "Green"=223, "Blue"=223}, {"Red"=224, "Green"=224, "Blue"=224}, {"Red"=225, "Green"=225, "Blue"=225}, {"Red"=226, "Green"=226, "Blue"=226}, {"Red"=227, "Green"=227, "Blue"=227}, {"Red"=228, "Green"=228, "Blue"=228}, {"Red"=229, "Green"=229, "Blue"=229}, {"Red"=230, "Green"=230, "Blue"=230}, {"Red"=231, "Green"=231, "Blue"=231}, {"Red"=232, "Green"=232, "Blue"=232}, {"Red"=233, "Green"=233, "Blue"=233}, {"Red"=234, "Green"=234, "Blue"=234}, {"Red"=235, "Green"=235, "Blue"=235}, {"Red"=236, "Green"=236, "Blue"=236}, {"Red"=237, "Green"=237, "Blue"=237}, {"Red"=238, "Green"=238, "Blue"=238}, {"Red"=239, "Green"=239, "Blue"=239}, {"Red"=240, "Green"=240, "Blue"=240}, {"Red"=241, "Green"=241, "Blue"=241}, {"Red"=242, "Green"=242, "Blue"=242}, {"Red"=243, "Green"=243, "Blue"=243}, {"Red"=244, "Green"=244, "Blue"=244}, {"Red"=245, "Green"=245, "Blue"=245}, {"Red"=246, "Green"=246, "Blue"=246}, {"Red"=247, "Green"=247, "Blue"=247}, {"Red"=248, "Green"=248, "Blue"=248}, {"Red"=249, "Green"=249, "Blue"=249}, {"Red"=250, "Green"=250, "Blue"=250}, {"Red"=251, "Green"=251, "Blue"=251}, {"Red"=252, "Green"=252, "Blue"=252}, {"Red"=253, "Green"=253, "Blue"=253}, {"Red"=254, "Green"=254, "Blue"=254}, {"Red"=255, "Green"=0, "Blue"=0}] ("Color Palette") cluster{"Red":u8, "Green":u8, "Blue":u8}[] [{"Red"=0, "Green"=0, "Blue"=0}, {"Red"=1, "Green"=1, "Blue"=1}, {"Red"=2, "Green"=2, "Blue"=2}, {"Red"=3, "Green"=3, "Blue"=3}, {"Red"=4, "Green"=4, "Blue"=4}, {"Red"=5, "Green"=5, "Blue"=5}, {"Red"=6, "Green"=6, "Blue"=6}, {"Red"=7, "Green"=7, "Blue"=7}, {"Red"=8, "Green"=8, "Blue"=8}, {"Red"=9, "Green"=9, "Blue"=9}, {"Red"=10, "Green"=10, "Blue"=10}, {"Red"=11, "Green"=11, "Blue"=11}, {"Red"=12, "Green"=12, "Blue"=12}, {"Red"=13, "Green"=13, "Blue"=13}, {"Red"=14, "Green"=14, "Blue"=14}, {"Red"=15, "Green"=15, "Blue"=15}, {"Red"=16, "Green"=16, "Blue"=16}, {"Red"=17, "Green"=17, "Blue"=17}, {"Red"=18, "Green"=18, "Blue"=18}, {"Red"=19, "Green"=19, "Blue"=19}, {"Red"=20, "Green"=20, "Blue"=20}, {"Red"=21, "Green"=21, "Blue"=21}, {"Red"=22, "Green"=22, "Blue"=22}, {"Red"=23, "Green"=23, "Blue"=23}, {"Red"=24, "Green"=24, "Blue"=24}, {"Red"=25, "Green"=25, "Blue"=25}, {"Red"=26, "Green"=26, "Blue"=26}, {"Red"=27, "Green"=27, "Blue"=27}, {"Red"=28, "Green"=28, "Blue"=28}, {"Red"=29, "Green"=29, "Blue"=29}, {"Red"=30, "Green"=30, "Blue"=30}, {"Red"=31, "Green"=31, "Blue"=31}, {"Red"=32, "Green"=32, "Blue"=32}, {"Red"=33, "Green"=33, "Blue"=33}, {"Red"=34, "Green"=34, "Blue"=34}, {"Red"=35, "Green"=35, "Blue"=35}, {"Red"=36, "Green"=36, "Blue"=36}, {"Red"=37, "Green"=37, "Blue"=37}, {"Red"=38, "Green"=38, "Blue"=38}, {"Red"=39, "Green"=39, "Blue"=39}, {"Red"=40, "Green"=40, "Blue"=40}, {"Red"=41, "Green"=41, "Blue"=41}, {"Red"=42, "Green"=42, "Blue"=42}, {"Red"=43, "Green"=43, "Blue"=43}, {"Red"=44, "Green"=44, "Blue"=44}, {"Red"=45, "Green"=45, "Blue"=45}, {"Red"=46, "Green"=46, "Blue"=46}, {"Red"=47, "Green"=47, "Blue"=47}, {"Red"=48, "Green"=48, "Blue"=48}, {"Red"=49, "Green"=49, "Blue"=49}, {"Red"=50, "Green"=50, "Blue"=50}, {"Red"=51, "Green"=51, "Blue"=51}, {"Red"=52, "Green"=52, "Blue"=52}, {"Red"=53, "Green"=53, "Blue"=53}, {"Red"=54, "Green"=54, "Blue"=54}, {"Red"=55, "Green"=55, "Blue"=55}, {"Red"=56, "Green"=56, "Blue"=56}, {"Red"=57, "Green"=57, "Blue"=57}, {"Red"=58, "Green"=58, "Blue"=58}, {"Red"=59, "Green"=59, "Blue"=59}, {"Red"=60, "Green"=60, "Blue"=60}, {"Red"=61, "Green"=61, "Blue"=61}, {"Red"=62, "Green"=62, "Blue"=62}, {"Red"=63, "Green"=63, "Blue"=63}, {"Red"=64, "Green"=64, "Blue"=64}, {"Red"=65, "Green"=65, "Blue"=65}, {"Red"=66, "Green"=66, "Blue"=66}, {"Red"=67, "Green"=67, "Blue"=67}, {"Red"=68, "Green"=68, "Blue"=68}, {"Red"=69, "Green"=69, "Blue"=69}, {"Red"=70, "Green"=70, "Blue"=70}, {"Red"=71, "Green"=71, "Blue"=71}, {"Red"=72, "Green"=72, "Blue"=72}, {"Red"=73, "Green"=73, "Blue"=73}, {"Red"=74, "Green"=74, "Blue"=74}, {"Red"=75, "Green"=75, "Blue"=75}, {"Red"=76, "Green"=76, "Blue"=76}, {"Red"=77, "Green"=77, "Blue"=77}, {"Red"=78, "Green"=78, "Blue"=78}, {"Red"=79, "Green"=79, "Blue"=79}, {"Red"=80, "Green"=80, "Blue"=80}, {"Red"=81, "Green"=81, "Blue"=81}, {"Red"=82, "Green"=82, "Blue"=82}, {"Red"=83, "Green"=83, "Blue"=83}, {"Red"=84, "Green"=84, "Blue"=84}, {"Red"=85, "Green"=85, "Blue"=85}, {"Red"=86, "Green"=86, "Blue"=86}, {"Red"=87, "Green"=87, "Blue"=87}, {"Red"=88, "Green"=88, "Blue"=88}, {"Red"=89, "Green"=89, "Blue"=89}, {"Red"=90, "Green"=90, "Blue"=90}, {"Red"=91, "Green"=91, "Blue"=91}, {"Red"=92, "Green"=92, "Blue"=92}, {"Red"=93, "Green"=93, "Blue"=93}, {"Red"=94, "Green"=94, "Blue"=94}, {"Red"=95, "Green"=95, "Blue"=95}, {"Red"=96, "Green"=96, "Blue"=96}, {"Red"=97, "Green"=97, "Blue"=97}, {"Red"=98, "Green"=98, "Blue"=98}, {"Red"=99, "Green"=99, "Blue"=99}, {"Red"=100, "Green"=100, "Blue"=100}, {"Red"=101, "Green"=101, "Blue"=101}, {"Red"=102, "Green"=102, "Blue"=102}, {"Red"=103, "Green"=103, "Blue"=103}, {"Red"=104, "Green"=104, "Blue"=104}, {"Red"=105, "Green"=105, "Blue"=105}, {"Red"=106, "Green"=106, "Blue"=106}, {"Red"=107, "Green"=107, "Blue"=107}, {"Red"=108, "Green"=108, "Blue"=108}, {"Red"=109, "Green"=109, "Blue"=109}, {"Red"=110, "Green"=110, "Blue"=110}, {"Red"=111, "Green"=111, "Blue"=111}, {"Red"=112, "Green"=112, "Blue"=112}, {"Red"=113, "Green"=113, "Blue"=113}, {"Red"=114, "Green"=114, "Blue"=114}, {"Red"=115, "Green"=115, "Blue"=115}, {"Red"=116, "Green"=116, "Blue"=116}, {"Red"=117, "Green"=117, "Blue"=117}, {"Red"=118, "Green"=118, "Blue"=118}, {"Red"=119, "Green"=119, "Blue"=119}, {"Red"=120, "Green"=120, "Blue"=120}, {"Red"=121, "Green"=121, "Blue"=121}, {"Red"=122, "Green"=122, "Blue"=122}, {"Red"=123, "Green"=123, "Blue"=123}, {"Red"=124, "Green"=124, "Blue"=124}, {"Red"=125, "Green"=125, "Blue"=125}, {"Red"=126, "Green"=126, "Blue"=126}, {"Red"=127, "Green"=127, "Blue"=127}, {"Red"=128, "Green"=128, "Blue"=128}, {"Red"=129, "Green"=129, "Blue"=129}, {"Red"=130, "Green"=130, "Blue"=130}, {"Red"=131, "Green"=131, "Blue"=131}, {"Red"=132, "Green"=132, "Blue"=132}, {"Red"=133, "Green"=133, "Blue"=133}, {"Red"=134, "Green"=134, "Blue"=134}, {"Red"=135, "Green"=135, "Blue"=135}, {"Red"=136, "Green"=136, "Blue"=136}, {"Red"=137, "Green"=137, "Blue"=137}, {"Red"=138, "Green"=138, "Blue"=138}, {"Red"=139, "Green"=139, "Blue"=139}, {"Red"=140, "Green"=140, "Blue"=140}, {"Red"=141, "Green"=141, "Blue"=141}, {"Red"=142, "Green"=142, "Blue"=142}, {"Red"=143, "Green"=143, "Blue"=143}, {"Red"=144, "Green"=144, "Blue"=144}, {"Red"=145, "Green"=145, "Blue"=145}, {"Red"=146, "Green"=146, "Blue"=146}, {"Red"=147, "Green"=147, "Blue"=147}, {"Red"=148, "Green"=148, "Blue"=148}, {"Red"=149, "Green"=149, "Blue"=149}, {"Red"=150, "Green"=150, "Blue"=150}, {"Red"=151, "Green"=151, "Blue"=151}, {"Red"=152, "Green"=152, "Blue"=152}, {"Red"=153, "Green"=153, "Blue"=153}, {"Red"=154, "Green"=154, "Blue"=154}, {"Red"=155, "Green"=155, "Blue"=155}, {"Red"=156, "Green"=156, "Blue"=156}, {"Red"=157, "Green"=157, "Blue"=157}, {"Red"=158, "Green"=158, "Blue"=158}, {"Red"=159, "Green"=159, "Blue"=159}, {"Red"=160, "Green"=160, "Blue"=160}, {"Red"=161, "Green"=161, "Blue"=161}, {"Red"=162, "Green"=162, "Blue"=162}, {"Red"=163, "Green"=163, "Blue"=163}, {"Red"=164, "Green"=164, "Blue"=164}, {"Red"=165, "Green"=165, "Blue"=165}, {"Red"=166, "Green"=166, "Blue"=166}, {"Red"=167, "Green"=167, "Blue"=167}, {"Red"=168, "Green"=168, "Blue"=168}, {"Red"=169, "Green"=169, "Blue"=169}, {"Red"=170, "Green"=170, "Blue"=170}, {"Red"=171, "Green"=171, "Blue"=171}, {"Red"=172, "Green"=172, "Blue"=172}, {"Red"=173, "Green"=173, "Blue"=173}, {"Red"=174, "Green"=174, "Blue"=174}, {"Red"=175, "Green"=175, "Blue"=175}, {"Red"=176, "Green"=176, "Blue"=176}, {"Red"=177, "Green"=177, "Blue"=177}, {"Red"=178, "Green"=178, "Blue"=178}, {"Red"=179, "Green"=179, "Blue"=179}, {"Red"=180, "Green"=180, "Blue"=180}, {"Red"=181, "Green"=181, "Blue"=181}, {"Red"=182, "Green"=182, "Blue"=182}, {"Red"=183, "Green"=183, "Blue"=183}, {"Red"=184, "Green"=184, "Blue"=184}, {"Red"=185, "Green"=185, "Blue"=185}, {"Red"=186, "Green"=186, "Blue"=186}, {"Red"=187, "Green"=187, "Blue"=187}, {"Red"=188, "Green"=188, "Blue"=188}, {"Red"=189, "Green"=189, "Blue"=189}, {"Red"=190, "Green"=190, "Blue"=190}, {"Red"=191, "Green"=191, "Blue"=191}, {"Red"=192, "Green"=192, "Blue"=192}, {"Red"=193, "Green"=193, "Blue"=193}, {"Red"=194, "Green"=194, "Blue"=194}, {"Red"=195, "Green"=195, "Blue"=195}, {"Red"=196, "Green"=196, "Blue"=196}, {"Red"=197, "Green"=197, "Blue"=197}, {"Red"=198, "Green"=198, "Blue"=198}, {"Red"=199, "Green"=199, "Blue"=199}, {"Red"=200, "Green"=200, "Blue"=200}, {"Red"=201, "Green"=201, "Blue"=201}, {"Red"=202, "Green"=202, "Blue"=202}, {"Red"=203, "Green"=203, "Blue"=203}, {"Red"=204, "Green"=204, "Blue"=204}, {"Red"=205, "Green"=205, "Blue"=205}, {"Red"=206, "Green"=206, "Blue"=206}, {"Red"=207, "Green"=207, "Blue"=207}, {"Red"=208, "Green"=208, "Blue"=208}, {"Red"=209, "Green"=209, "Blue"=209}, {"Red"=210, "Green"=210, "Blue"=210}, {"Red"=211, "Green"=211, "Blue"=211}, {"Red"=212, "Green"=212, "Blue"=212}, {"Red"=213, "Green"=213, "Blue"=213}, {"Red"=214, "Green"=214, "Blue"=214}, {"Red"=215, "Green"=215, "Blue"=215}, {"Red"=216, "Green"=216, "Blue"=216}, {"Red"=217, "Green"=217, "Blue"=217}, {"Red"=218, "Green"=218, "Blue"=218}, {"Red"=219, "Green"=219, "Blue"=219}, {"Red"=220, "Green"=220, "Blue"=220}, {"Red"=221, "Green"=221, "Blue"=221}, {"Red"=222, "Green"=222, "Blue"=222}, {"Red"=223, "Green"=223, "Blue"=223}, {"Red"=224, "Green"=224, "Blue"=224}, {"Red"=225, "Green"=225, "Blue"=225}, {"Red"=226, "Green"=226, "Blue"=226}, {"Red"=227, "Green"=227, "Blue"=227}, {"Red"=228, "Green"=228, "Blue"=228}, {"Red"=229, "Green"=229, "Blue"=229}, {"Red"=230, "Green"=230, "Blue"=230}, {"Red"=231, "Green"=231, "Blue"=231}, {"Red"=232, "Green"=232, "Blue"=232}, {"Red"=233, "Green"=233, "Blue"=233}, {"Red"=234, "Green"=234, "Blue"=234}, {"Red"=235, "Green"=235, "Blue"=235}, {"Red"=236, "Green"=236, "Blue"=236}, {"Red"=237, "Green"=237, "Blue"=237}, {"Red"=238, "Green"=238, "Blue"=238}, {"Red"=239, "Green"=239, "Blue"=239}, {"Red"=240, "Green"=240, "Blue"=240}, {"Red"=241, "Green"=241, "Blue"=241}, {"Red"=242, "Green"=242, "Blue"=242}, {"Red"=243, "Green"=243, "Blue"=243}, {"Red"=244, "Green"=244, "Blue"=244}, {"Red"=245, "Green"=245, "Blue"=245}, {"Red"=246, "Green"=246, "Blue"=246}, {"Red"=247, "Green"=247, "Blue"=247}, {"Red"=248, "Green"=248, "Blue"=248}, {"Red"=249, "Green"=249, "Blue"=249}, {"Red"=250, "Green"=250, "Blue"=250}, {"Red"=251, "Green"=251, "Blue"=251}, {"Red"=252, "Green"=252, "Blue"=252}, {"Red"=253, "Green"=253, "Blue"=253}, {"Red"=254, "Green"=254, "Blue"=254}, {"Red"=255, "Green"=255, "Blue"=255}] ("Color Palette")] -> w151
              frame "high clipping red" {
              }
              frame "low clipping blue" {
              }
              frame "high and low clipping" {
              }
              frame "standard", "high / low (full range)" {
              }
            }
            n89 = call-poly "GFGpolyGet.vi"() -> ("error out"=w156:errorcluster, "DisplayRefsOut(generic class)"=w155:T12)  [unwired: 10 in]
            n90 = Cluster To Array(cluster=w155) -> (array=w153:refnum<vi>[])
            n91 = for {
              tunnel: w153 -> [w166] mode=indexing
              tunnel: w151 -> [w161]
              tunnel: w152 -> [w162]
              tunnel: w156 -> [w163]
              tunnel: w154 -> [w165]
              n92 = To More Specific Class(target class=w165, reference=w166) -> (specific class reference=w164:refnum<vi>)  [unwired: 1 in, 1 out]
              n93 = property class="ImageControl"(reference=w164, error in=w163, "User Palette"=w161, "Palette Type"=w162) -> ()  [unwired: 2 out]
            }
          }
          frame "no..of.frames.to.acquire" {
            n94 = feedback #1() -> (w173:variant)  [unwired: 1 in]
            n95 = feedback-in #1(w171) -> ()
            n96 = Variant To Data(type=0.0, Variant=w171) -> (data=w178:dbl)  [unwired: 1 in, 1 out]
            n97 = Not Equal?(x=w171, y=w173) -> (x != y?=w172:bool)
            n98 = case shown="True" w172 {
              frame False {
              }
              frame True {
                n99 = call "calculate tiff files size.vi"() -> ()  [unwired: 11 in, 1 out]
              }
            }
            n100 = call-poly "GFGpolyGet.vi"("Variable Name in"="frame count") -> ("output cluster"=w188:T2)  [unwired: 9 in, 1 out]
            n101 = call-poly "GFGpolyGet.vi"("Variable Name in"="frames.per.z.cycle") -> ("Numeric"=w177:dbl)  [unwired: 8 in, 2 out]
            n102 = call "GFG_core.vi"("Variable Name in"="scan mode main settings") -> ("Variant Out"=w183:variant)  [unwired: 12 in, 6 out]
            n103 = Variant To Data(type=scan_mode_main_settings_tab."2D line scan" ("scan mode main settings"), Variant=w183) -> (data=w181:T4)  [unwired: 1 in, 1 out]
            n104 = Unbundle By Name(w188) -> ("SlideRef"=w187:refnum<vi>)
            n105 = property class="Slide"(reference=w187, "Scale.Maximum"=w178) -> ()  [unwired: 1 in, 2 out]
            n106 = case shown="\"2D frame\", Default" w181 {
              tunnel: w178 -> [w190 _]
              frame "2D frame", Default {
                n107 = call "GFG_core.vi"("Variable Name in"="no.of.frames.for.frame.scan", "Variant in"=w190, "Action"=enum16{"Init", "Set", "Get"}."Set") -> ()  [unwired: 10 in, 7 out]
              }
              frame "2D line scan" {
              }
            }
            n108 = Divide(x=w178, y=w177) -> (x/y=w174:dbl)
            n109 = call "GFG_core.vi"("Variable Name in"="no.of.cycles.to.scan", "Variant in"=w174, "Action"=enum16{"Init", "Set", "Get", "Clear"}."Set") -> ()  [unwired: 10 in, 7 out]
          }
          frame "frames.per.z.cycle", "no.of.cycles.to.scan" {
            n110 = call "getVIname.vi"() -> ("VI name"=w199:string)  [unwired: 19 in]
            n111 = Not Equal?(x=w193, y=w199) -> (x != y?=w198:bool)
            n112 = call-poly "GFGpolyGet.vi"("Variable Name in"="frames.p.sec") -> ("Numeric"=w196:dbl)  [unwired: 8 in, 2 out]
            n113 = call-poly "GFGpolyGet.vi"("Variable Name in"="frames.per.z.cycle") -> ("Numeric"=w195:dbl)  [unwired: 8 in, 2 out]
            n114 = Divide(x=w196, y=w195) -> (x/y=w194:dbl)
            n115 = call "GFG_core.vi"("Variable Name in"="volume rate (in Hz)", "Variant in"=w194, "Action"=enum16{"Init", "Set", "Get", "Clear"}."Set") -> ()  [unwired: 10 in, 7 out]
            n116 = case shown="True" w198 {
              tunnel: w195 -> [_ w216]
              frame False {
              }
              frame True {
                n117 = call-poly "GFGpolyGet.vi"("Variable Name in"="no.of.cycles.to.scan") -> ("Numeric"=w209:dbl)  [unwired: 8 in, 2 out]
                n118 = call-poly "GFGpolyGet.vi"("Variable Name in"="frames.p.queue.item") -> ("Numeric"=w214:dbl)  [unwired: 8 in, 2 out]
                n119 = feedback #2() -> (w208:dbl)  [unwired: 1 in]
                n120 = Greater?(x=w208, y=w209) -> (0:w206:bool)
                n121 = while {
                  tunnel: w216 -> [w226]
                  shift-right: [w223] -> w205
                  shift-left: w209 -> [w220]
                  tunnel: w214 -> [w225]
                  tunnel: [w222] -> w207
                  tunnel: w206 -> [w218]
                  stop <- w221 stop-if-true
                  n122 = Multiply(x=w226, y=w220) -> (x*y=w222:dbl)
                  n123 = Round Toward +Infinity(x=w220) -> (ceil(x): smallest int >= x=w219:dbl)
                  n124 = Quotient & Remainder(x=w222, y=w225) -> (x-y*floor(x/y)=w224:dbl)  [unwired: 1 out]
                  n125 = Equal To 0?(x=w224) -> (x = 0?=w221:bool)
                  n126 = case shown="False" w221 {
                    tunnel: w219 -> [w231 w232]
                    tunnel: [w227 w232] -> w223
                    tunnel: w218 -> [w228 _]
                    frame False {
                      n127 = Decrement(x=w231) -> (x-1=w230:dbl)
                      n128 = Increment(x=w231) -> (x+1=w229:dbl)
                      n129 = Select(t=w230, s=w228, f=w229) -> (s? t:f=w227:dbl)
                    }
                    frame True {
                    }
                  }
                }
                n130 = feedback-in #2(w205) -> ()
                n131 = call "GFG_core.vi"("Variable Name in"="no. of frames to acquire", "Variant in"=w207, "Action"=enum16{"Init", "Set", "Get", "Clear"}."Set") -> ()  [unwired: 10 in, 7 out]
                n132 = call "GFG_core.vi"("Variable Name in"="no.of.cycles.to.scan", "Variant in"=w205, "Action"=enum16{"Init", "Set", "Get", "Clear"}."Set") -> ()  [unwired: 10 in, 7 out]
              }
            }
          }
          frame "Start.Delay", "ZOOM", "invert.ch.1", "invert.ch.2", "invert.ch.3", "invert.ch.4", "pixel.resolution", "speed.mode" {
            n133 = Equal?(x=w234, y="fp button handler_crMD.vi") -> (x = y?=w236:bool)
            n134 = Equal?(x=w234, y="start_delay_autocorrect_rrMD.vi") -> (x = y?=w238:bool)
            n135 = Equal?(x=w234, y="calculation.vi mouse event" ("Source VI")) -> (x = y?=w240:bool)
            n136 = Compound Arithmetic op=OR(w236, w238, w240) -> (w233:bool)
            n137 = flat-sequence {
              tunnel: w245 -> [w247]
              tunnel: w244 -> [w255]
              tunnel: w243 -> [w253]
              tunnel: w241 -> [w251]
              tunnel: w233 -> [w250]
              tunnel: w234 -> [w249]
              frame #0 {
                n138 = case shown="True" w250 {
                  tunnel: w247 -> [_ w380]
                  tunnel: [_ w379] -> w254
                  tunnel: w251 -> [_ w378]
                  tunnel: w249 -> [_ w377]
                  frame False {
                  }
                  frame True {
                    n139 = flat-sequence {
                      tunnel: w380 -> [w387]
                      tunnel: [w388] -> w382
                      tunnel: w378 -> [w388]
                      tunnel: [w384] -> w381
                      tunnel: w377 -> [w383]
                      tunnel: [w383] -> w376
                      tunnel: [w411] -> w379
                      tunnel: w382 -> [w410]
                      tunnel: w381 -> [w409]
                      tunnel: w376 -> [w408]
                      frame #0 {
                        n140 = call "Timer.vi"("Timer Command"=Timer_Commands."Check Time", "name qualifier (empty if unwired)"="flystop censor period") -> ("Complete?"=w384:bool)  [unwired: 4 in, 5 out]
                        n141 = case shown="True" w384 {
                          tunnel: w387 -> [_ w389]
                          frame False {
                          }
                          frame True {
                            n142 = call-poly "GFGpolyGet.vi"("Variable Name in"=w389) -> ("output cluster"=w404:T2)  [unwired: 9 in, 1 out]
                            n143 = Unbundle(w404) -> ("WaveformChartRef"=w400:refnum<vi>, "DigitalRef"=w399:refnum<vi>, "ArrayRef"=w398:refnum<vi>, "TabControlRef"=w397:refnum<vi>, "EnumRef"=w396:refnum<vi>, "RingRef"=w395:refnum<vi>, "BooleanRef"=w394:refnum<vi>, "KnobRef"=w393:refnum<vi>, "SlideRef"=w392:refnum<vi>, "PathRef"=w391:refnum<vi>, "StringRef"=w390:refnum<vi>, "ComboBox"=w401:refnum<vi>, "WaveformGraphRef"=w402:refnum<vi>)
                            n144 = Build Array(w400, w399, w398, w397, w396, w395, w394, w393, w392, w391, w390, w401, w402) -> (w403:refnum<vi>[])
                            n145 = for {
                              tunnel: w403 -> [w406] mode=indexing
                              tunnel: [w406] -> w405
                              stop <- w407 continue-if-true
                              n146 = Not A Number/Path/Refnum?(number/path/refnum=w406) -> (NaN/Path/Refnum?=w407:bool)
                            }
                            n147 = call "wait for fp element value stable.vi"("CtlRef"=w405) -> ()  [unwired: 9 in, 2 out]
                          }
                        }
                      }
                      frame #1 {
                        n148 = case shown="True" w409 {
                          tunnel: [_ w418] -> w411
                          tunnel: w410 -> [_ w417]
                          tunnel: w408 -> [_ w412]
                          frame False {
                          }
                          frame True {
                            n149 = call-poly "GFGpolyGet.vi"("Variable Name in"="FOCUS") -> ("Boolean Value OUT"=w413:bool)  [unwired: 9 in, 1 out]
                            n150 = call "GFG_core.vi"("Variable Name in"="flystop", "Variant in"=w413, "Action"=enum16{"Init", "Set", "Get"}."Set") -> ("error out"=w418:errorcluster)  [unwired: 10 in, 6 out]
                            n151 = case shown="True" w413 {
                              tunnel: w417 -> [_ _]
                              tunnel: w412 -> [w419 _]
                              frame True {
                                n152 = Build Array("Start.Delay" ("Variable Name in"), "ZOOM" ("Variable Name in"), "x.correction" ("Variable Name in")) -> (w426:string[])
                                n153 = for {
                                tunnel: w426 -> [w427] mode=indexing
                                n154 = call-poly "GFGpolyGet.vi"("Variable Name in"=w427) -> ("output cluster"=w430:T2)  [unwired: 9 in, 1 out]
                                n155 = Unbundle By Name(w430) -> ("SlideRef"=w428:refnum<vi>)
                                n156 = property class="Slide"(reference=w428, "DisabledEnum"=T5."Disabled and Grayed Out" ("Disabled")) -> ()  [unwired: 1 in, 2 out]
                                }
                                n157 = call "Timer.vi"("Timer Command"=Timer_Commands."Start", "name qualifier (empty if unwired)"="flystop censor period", "Set Time IN (s)"=5.0) -> ()  [unwired: 3 in, 6 out]
                                "Source VI 2" <- w419
                              }
                              frame False {
                                n158 = Build Array("Start.Delay" ("Variable Name in"), "ZOOM" ("Variable Name in"), "x.correction" ("Variable Name in")) -> (w434:string[])
                                n159 = for {
                                tunnel: w434 -> [w435] mode=indexing
                                n160 = call-poly "GFGpolyGet.vi"("Variable Name in"=w435) -> ("output cluster"=w438:T2)  [unwired: 9 in, 1 out]
                                n161 = Unbundle By Name(w438) -> ("SlideRef"=w436:refnum<vi>)
                                n162 = property class="Slide"(reference=w436, "DisabledEnum"=T5."Enabled" ("Disabled")) -> ()  [unwired: 1 in, 2 out]
                                }
                              }
                            }
                          }
                        }
                      }
                    }
                  }
                }
                n163 = flat-sequence {
                  tunnel: [w261] -> w256
                  tunnel: w247 -> [w260]
                  tunnel: w255 -> [w259]
                  tunnel: w254 -> [w258]
                  tunnel: [w257] -> w252
                  frame #0 {
                    n164 = case shown="\"ZOOM\", Default" w260 {
                      tunnel: w259 -> [_ _ _ w292]
                      tunnel: [w263 w273 w284 w294] -> w261
                      tunnel: w258 -> [_ _ _ _]
                      tunnel: [_ _ _ w290] -> w257
                      frame "ZOOM", Default {
                        w262 = pixel_resolution_resonant_enum."512 x  64"  # pixel resolution
                        n165 = call "GFG_core.vi"("Variable Name in"="pixel.resolution") -> ("Variant Out"=w264:variant)  [unwired: 12 in, 6 out]
                        n166 = Variant To Data(type=w262, Variant=w264) -> (data=w263:T13)  [unwired: 1 in, 1 out]
                      }
                      frame "x.correction" {
                        w272 = pixel_resolution_resonant_enum."512 x 512"  # pixel resolution
                        n167 = call-poly "GFGpolyGet.vi"("Variable Name in"="resonant.correction.enable") -> ("Boolean Value OUT"=w269:bool)  [unwired: 9 in, 1 out]
                        n168 = call-poly "GFGpolyGet.vi"("Variable Name in"="x.correction") -> ("Numeric"=w266:dbl)  [unwired: 8 in, 2 out]
                        n169 = call "GFG_core.vi"("Variable Name in"="pixel.resolution") -> ("Variant Out"=w274:variant)  [unwired: 12 in, 6 out]
                        n170 = case shown="True" w269 {
                          tunnel: ["x.correction.shift" ("Variable Name in") "x.correction.cosine" ("Variable Name in")] -> w267
                          frame False {
                          }
                          frame True {
                          }
                        }
                        n171 = Variant To Data(type=w272, Variant=w274) -> (data=w273:T13)  [unwired: 1 in, 1 out]
                        n172 = call "GFG_core.vi"("Variable Name in"=w267, "Variant in"=w266, "Action"=enum16{"Init", "Set", "Get"}."Set") -> ()  [unwired: 10 in, 7 out]
                      }
                      frame "resonant.correction.enable" {
                        w278 = pixel_resolution_resonant_enum."512 x 512"  # pixel resolution
                        n173 = call-poly "GFGpolyGet.vi"("Variable Name in"="resonant.correction.enable") -> ("Boolean Value OUT"=w283:bool)  [unwired: 9 in, 1 out]
                        n174 = call "GFG_core.vi"("Variable Name in"="pixel.resolution") -> ("Variant Out"=w285:variant)  [unwired: 12 in, 6 out]
                        n175 = case shown="True" w283 {
                          tunnel: ["x.correction.shift" ("Variable Name in") "x.correction.cosine" ("Variable Name in")] -> w280
                          frame False {
                          }
                          frame True {
                          }
                        }
                        n176 = Variant To Data(type=w278, Variant=w285) -> (data=w284:T13)  [unwired: 1 in, 1 out]
                        n177 = call-poly "GFGpolyGet.vi"("Variable Name in"=w280) -> ("Numeric"=w281:dbl)  [unwired: 8 in, 2 out]
                        n178 = call "GFG_core.vi"("Variable Name in"="x.correction", "Variant in"=w281, "Action"=enum16{"Init", "Set", "Get"}."Set") -> ()  [unwired: 10 in, 7 out]
                      }
                      frame "pixel.resolution" {
                        w293 = pixel_resolution_resonant_enum."512 x 512"  # pixel resolution
                        n179 = Variant To Data(type=w293, Variant=w292) -> (data=w294:T13)  [unwired: 1 in, 1 out]
                        n180 = feedback-in #3(w292) -> ()
                        n181 = feedback #3() -> (w291:variant)  [unwired: 1 in]
                        n182 = Not Equal?(x=w292, y=w291) -> (x != y?=w290:bool)
                      }
                    }
                  }
                }
                n183 = flat-sequence {
                  tunnel: w256 -> [w303]
                  tunnel: w253 -> [w345]
                  tunnel: w252 -> [w297]
                  tunnel: [w297] -> w248
                  tunnel: w248 -> [w375]
                  frame #0 {
                    n184 = case shown="\"512 x arbitrary\", \" 1024 x arbitrary\", \" 1536 x arbitrary\"" w303 {
                      tunnel: [T5."Disabled and Grayed Out" ("Disabled") T5."Enabled" ("Disabled")] -> w299
                      frame Default {
                      }
                      frame "512 x arbitrary", " 1024 x arbitrary", " 1536 x arbitrary" {
                      }
                    }
                    n185 = call "check hardware configuration.vi"() -> ("bitfile name"=w307:T14)  [unwired: 7 in, 4 out]
                    n186 = call "GFG_core.vi"("Variable Name in"="MAIN.Image.panels.reso.") -> ("Variant Out"=w314:variant)  [unwired: 12 in, 6 out]
                    n187 = Build Array("nomin.x.pixels" ("Variable Name in"), "y.pixel.sz" ("Variable Name in"), "x.pixel.sz" ("Variable Name in")) -> (w339:string[])
                    n188 = call "GFG_core.vi"("Variable Name in"="bitfile.name", "Variant in"=w307, "Action"=enum16{"Init", "Set", "Get"}."Set") -> ()  [unwired: 10 in, 7 out]
                    n189 = Variant To Data(type=MAIN_Image_panel_reso_tab_Control_type_def."Channel 2" ("MAIN Image panels reso"), Variant=w314) -> (data=w312:T6)  [unwired: 1 in, 1 out]
                    n190 = call-poly "GFGpolyGet.vi"("Variable Name in"="y.pixels") -> ("output cluster"=w301:T2)  [unwired: 9 in, 1 out]
                    n191 = for {
                      tunnel: w339 -> [w374] mode=indexing
                      tunnel: T5."Disabled and Grayed Out" ("Disabled") -> [w371]
                      n192 = call-poly "GFGpolyGet.vi"("Variable Name in"=w374) -> ("output cluster"=w373:T2)  [unwired: 9 in, 1 out]
                      n193 = Unbundle By Name(w373) -> ("DigitalRef"=w372:refnum<vi>)
                      n194 = property class="DigNum"(reference=w372, "DisabledEnum"=w371) -> ()  [unwired: 1 in, 2 out]
                    }
                    n195 = Unbundle By Name(w301) -> ("DigitalRef"=w300:refnum<vi>)
                    n196 = Less?(x=w312, y=MAIN_Image_panel_reso_tab_Control_type_def."Channel 5") -> (x < y?=w310:bool)
                    n197 = case shown="\"512 x arbitrary\"" w303 {
                      tunnel: [512 512 512 512 1024 1024 1536 1536 512 1024] -> w295
                      tunnel: [64 128 256 512 512 1024 512 w362 w365 w368] -> w319
                      tunnel: w310 -> [_ _ _ _ _ _ _ _ _ _]
                      frame "512 x  64" {
                      }
                      frame "512 x 128" {
                      }
                      frame "512 x 256" {
                      }
                      frame "512 x 512", Default {
                      }
                      frame "1024 x 512" {
                      }
                      frame "1024 x 1024" {
                      }
                      frame " 1536 x  512" {
                      }
                      frame " 1536 x arbitrary" {
                        n198 = call-poly "GFGpolyGet.vi"("Variable Name in"="y.pixels") -> ("Numeric"=w362:dbl)  [unwired: 8 in, 2 out]
                      }
                      frame "512 x arbitrary" {
                        n199 = call-poly "GFGpolyGet.vi"("Variable Name in"="y.pixels") -> ("Numeric"=w365:dbl)  [unwired: 8 in, 2 out]
                      }
                      frame " 1024 x arbitrary" {
                        n200 = call-poly "GFGpolyGet.vi"("Variable Name in"="y.pixels") -> ("Numeric"=w368:dbl)  [unwired: 8 in, 2 out]
                      }
                    }
                    n201 = property class="DigNum"(reference=w300, "DisabledEnum"=w299) -> ()  [unwired: 1 in, 2 out]
                    n202 = Select(t=11960, s=w345, f=7910) -> (s? t:f=w304:i32)
                    n203 = call "GFG_core.vi"("Variable Name in"="y.pixels", "Variant in"=w319, "Action"=enum16{"Init", "Set", "Get"}."Set") -> ()  [unwired: 10 in, 7 out]
                    n204 = Multiply(x=w304, y=2.0) -> (x*y=w320:dbl)
                    n205 = Divide(x=w320, y=w319) -> (x/y=w316:dbl)
                    n206 = call-poly "GFGpolyGet.vi"("Variable Name in"="max.field.of.view.resonant") -> ("Numeric"=w326:dbl)  [unwired: 8 in, 2 out]
                    n207 = call-poly "GFGpolyGet.vi"("Variable Name in"="max.field.of.view") -> ("Numeric"=w336:dbl)  [unwired: 8 in, 2 out]
                    n208 = call-poly "GFGpolyGet.vi"("Variable Name in"="ZOOM") -> ("Numeric"=w296:dbl)  [unwired: 8 in, 2 out]
                    n209 = call "GFG_core.vi"("Variable Name in"="frames.p.sec", "Variant in"=w316, "Action"=enum16{"Init", "Set", "Get"}."Set") -> ()  [unwired: 10 in, 7 out]
                    n210 = Divide(x=w326, y=w296) -> (x/y=w325:dbl)
                    n211 = Divide(x=w336, y=w296) -> (x/y=w329:dbl)
                    n212 = Divide(x=w325, y=w295) -> (x/y=w324:dbl)
                    n213 = Divide(x=w329, y=w295) -> (x/y=w328:dbl)
                    n214 = call "GFG_core.vi"("Variable Name in"="x.pixel.sz", "Variant in"=w324, "Action"=enum16{"Init", "Set", "Get"}."Set") -> ()  [unwired: 10 in, 7 out]
                    n215 = call "GFG_core.vi"("Variable Name in"="x.pixels", "Variant in"=w295, "Action"=enum16{"Init", "Set", "Get"}."Set") -> ()  [unwired: 10 in, 7 out]
                    n216 = call "GFG_core.vi"("Variable Name in"="nomin.x.pixels", "Variant in"=w295, "Action"=enum16{"Init", "Set", "Get"}."Set") -> ()  [unwired: 10 in, 7 out]
                    n217 = call "GFG_core.vi"("Variable Name in"="y.pixel.sz", "Variant in"=w328, "Action"=enum16{"Init", "Set", "Get"}."Set") -> ()  [unwired: 10 in, 7 out]
                  }
                  frame #1 {
                    n218 = case shown="True" w375 {
                      frame False {
                      }
                      frame True {
                        n219 = call "calculate tiff files size.vi"() -> ()  [unwired: 11 in, 1 out]
                      }
                    }
                  }
                }
              }
            }
          }
          frame "custom.step.xy", "custom.step.z" {
            n220 = Variant To Data(type=FALSE, Variant=w442) -> (data=w443:bool)  [unwired: 1 in, 1 out]
            n221 = case shown="True" w443 {
              tunnel: w441 -> [_ w446]
              frame False {
              }
              frame True {
                n222 = case shown="\"custom.step.xy\"" w446 {
                  tunnel: [w482 _ w484] -> w449
                  tunnel: ["step.size.z" ("Variable Name in") _ "step.size.xy" ("Variable Name in")] -> w454
                  frame "custom.step.z" {
                    n223 = call "Custom Step Size Z"() -> ("Custom Step Size Z"=w482:dbl)  [unwired: 17 in, 2 out]
                  }
                  frame Default {
                  }
                  frame "custom.step.xy" {
                    n224 = call "Custom Step Size XY"() -> ("Custom Step Size XY"=w484:dbl)  [unwired: 17 in, 2 out]
                  }
                }
                n225 = Equal?(x=w449, y=dbl[] [1.0, 2.0, 5.0, 10.0, 20.0, 50.0]) -> (x = y?=w452:bool[])
                n226 = Less Or Equal To 0?(x=w449) -> (x <= 0?=w447:bool)
                n227 = To Unsigned Word Integer(number=w449) -> (unsigned 16bit integer=w448:u16)
                n228 = Or Array Elements(Boolean array=w452) -> (logical OR=w451:bool)
                n229 = Or(x=w447, y=w451) -> (x .or. y?=w450:bool)
                n230 = case shown="True" w450 {
                  tunnel: w454 -> [w469 w473]
                  tunnel: w448 -> [w458 w472]
                  tunnel: w447 -> [_ w471]
                  tunnel: [w458 w470] -> w445
                  frame False {
                    n231 = call-poly "GFGpolyGet.vi"("Variable Name in"=w469) -> ("output cluster"=w468:T2)  [unwired: 9 in, 1 out]
                    n232 = Unbundle By Name(w468) -> ("RingRef"=w467:refnum<vi>)
                    n233 = property class="Ring"(reference=w467) -> (reference out=w462:refnum<vi>, "StringsAndValues[]"=w466:T15)  [unwired: 1 in, 1 out]
                    n234 = Number To Decimal String(number=w458) -> (decimal integer string=w464:string)  [unwired: 1 in]
                    n235 = Array Size(array=w466) -> (size(s)=w459:i32)
                    n236 = Decrement(x=w459) -> (x-1=w460:i32)
                    n237 = Index Array(array=w466, index=w460) -> (element=w465:cluster{"String":string, "Value":ext})
                    n238 = Bundle(cluster=w465, "String"=w464, "Value"=w458) -> (w463:cluster{"String":string, "Value":ext})
                    n239 = Replace Array Subset(array=w466, new element=w463, index=w460) -> (w461:T15)
                    n240 = property class="Ring"(reference=w462, "StringsAndValues[]"=w461, "Val(Sgnl)"=w458) -> ()  [unwired: 1 in, 2 out]
                  }
                  frame True {
                    # "Ignore values <=0 and standard values, as software would crash with duplicate entries. Entering 100 must be however still possible, as this is the last default value, which always will be repaced by the custom value. To reset it the input 100 must be allowed!"
                    n241 = Select(t=u16 0, s=w471, f=w472) -> (s? t:f=w474:u16)
                    n242 = case "Switch to existing value" shown="Default" w474 {
                      selector: w474 -> [w476 w478]
                      tunnel: [w476 w478] -> w470
                      tunnel: w473 -> [_ w477]
                      frame 0 {
                        # "Ignore values smaller or equal to zero"
                      }
                      frame Default {
                        n243 = call-poly "GFGpolyGet.vi"("Variable Name in"=w477) -> ("output cluster"=w480:T2)  [unwired: 9 in, 1 out]
                        n244 = Unbundle By Name(w480) -> ("RingRef"=w479:refnum<vi>)
                        n245 = property class="Ring"(reference=w479, "Val(Sgnl)"=w478) -> ()  [unwired: 1 in, 2 out]
                      }
                    }
                  }
                }
                n246 = flat-sequence {
                  tunnel: w446 -> [w456]
                  tunnel: w445 -> [_]
                  frame #0 {
                    n247 = call "GFG_core.vi"("Variable Name in"=w456, "Variant in"=FALSE, "Action"=enum16{"Init", "Set", "Get", "Clear"}."Set") -> ()  [unwired: 10 in, 7 out]
                  }
                }
              }
            }
          }
          frame "file.format", "save.ch.1", "save.ch.2", "save.ch.3", "save.ch.4" {
            n248 = case shown="\"save.ch.1\", \"save.ch.2\", \"save.ch.3\", \"save.ch.4\"" w485 {
              selector: w485 -> [w492 w498]
              tunnel: [w492 w497] -> w486
              frame Default {
              }
              frame "save.ch.1", "save.ch.2", "save.ch.3", "save.ch.4" {
                n249 = call-poly "GFGpolyGet.vi"("Variable Name in"="save.ch.1") -> ("Boolean Value OUT"=w496:bool)  [unwired: 9 in, 1 out]
                n250 = call-poly "GFGpolyGet.vi"("Variable Name in"="save.ch.2") -> ("Boolean Value OUT"=w495:bool)  [unwired: 9 in, 1 out]
                n251 = call-poly "GFGpolyGet.vi"("Variable Name in"="save.ch.3") -> ("Boolean Value OUT"=w494:bool)  [unwired: 9 in, 1 out]
                n252 = call-poly "GFGpolyGet.vi"("Variable Name in"="save.ch.4") -> ("Boolean Value OUT"=w493:bool)  [unwired: 9 in, 1 out]
                n253 = Boolean To (0,1)(Boolean=w496) -> (0, 1=w499:i16)
                n254 = Boolean To (0,1)(Boolean=w495) -> (0, 1=w500:i16)
                n255 = Boolean To (0,1)(Boolean=w494) -> (0, 1=w501:i16)
                n256 = Boolean To (0,1)(Boolean=w493) -> (0, 1=w502:i16)
                n257 = Compound Arithmetic op=ADD(w499, w500, w501, w502) -> (w503:i16)
                n258 = Equal To 0?(x=w503) -> (x = 0?=w504:bool)
                n259 = case shown="True" w504 {
                  tunnel: w498 -> [w509 w511]
                  tunnel: [w509 w511] -> w497
                  frame False {
                  }
                  frame True {
                    # "undo the change."
                    n260 = call "GFG_core.vi"("Variable Name in"=w511, "Variant in"=TRUE ("Value"), "Action"=enum16{"Init", "Set", "Get", "Clear"}."Set") -> ()  [unwired: 10 in, 7 out]
                    n261 = One Button Dialog(message="At least one channel must be selected! Please select another channel first to proceed!") -> ()  [unwired: 1 in, 1 out]
                  }
                }
              }
            }
            n262 = flat-sequence {
              tunnel: w486 -> [_]
              frame #0 {
                n263 = call "calculate tiff files size.vi"() -> ("no. of channels"=w489:i16)  [unwired: 11 in]
                n264 = call "GFG_core.vi"("Variable Name in"="no.of.channels" ("Tag in"), "Variant in"=w489, "Action"=enum16{"Init", "Set", "Get", "Clear"}."Set") -> ()  [unwired: 10 in, 7 out]
              }
            }
          }
          frame "reset.zoom" {
            n265 = call-poly "GFGpolyGet.vi"() -> ("DisplayRefsOut(generic class)"=w520:T12)  [unwired: 10 in, 1 out]
            n266 = call-poly "GFGpolyGet.vi"() -> ("Image Refs Out"=w519:T17)  [unwired: 10 in, 1 out]
            n267 = Cluster To Array(cluster=w520) -> (array=w518:refnum<vi>[])
            n268 = Cluster To Array(cluster=w519) -> (array=w517:T16[])
            n269 = call "set initial zoom.vi"("reset?"=TRUE, "Image Refs In"=w517, "DisplayRefsIn(generic class)"=w518) -> ()  [unwired: 9 in]
          }
          frame "max.field.of.view", "max.field.of.view.resonant", "nomin.x.pixels", "voltage.for.max.field.of.view", "voltage.for.max.field.of.view.resonant", "voltage.for.min.field.of.view.resonant", "x.pixel.sz", "x.volt.offset", "y.pixel.sz", "y.pixels", "y.volt.offset" {
            n270 = case shown="\"max.field.of.view\", \"max.field.of.view.resonant\", \"voltage.for.max.field.of.view\", \"voltage.for.max.field.of.view.resonant\", \"voltage.for.min.field.of.view.resonant\"" w521 {
              frame Default {
              }
              frame "max.field.of.view", "max.field.of.view.resonant", "voltage.for.max.field.of.view", "voltage.for.max.field.of.view.resonant", "voltage.for.min.field.of.view.resonant" {
                n271 = call-poly "GFGpolyGet.vi"("Variable Name in"="active.objective") -> ("Numeric"=w528:dbl)  [unwired: 8 in, 2 out]
                n272 = To Byte Integer(number=w528) -> (8bit integer=w526:i8)
                n273 = Increment(x=w526) -> (x+1=w529:i8)
                n274 = Number To Decimal String(number=w529) -> (decimal integer string=w527:string)  [unwired: 1 in]
                n275 = Build Array("max.field.of.view", "voltage.for.max.field.of.view", "max.field.of.view.resonant", "voltage.for.max.field.of.view.resonant", "voltage.for.min.field.of.view.resonant") -> (w533:string[])
                n276 = for {
                  tunnel: w533 -> [w544] mode=indexing
                  tunnel: w527 -> [w547]
                  tunnel: "obj" -> [w548]
                  tunnel: "." -> [w546]
                  n277 = Concatenate Strings(w548, w547, w546, w544) -> (w545:string)
                  n278 = Build Array(w545, w544) -> (w540:string[])
                  n279 = Reverse 1D Array(array=w540) -> (reversed array=w539:string[])
                  n280 = Build Array(enum16{"Init", "Set", "Get"}."Get" ("Action"), enum16{"Init", "Set", "Get"}."Set" ("Action")) -> (w541:enum16{"Init", "Set", "Get"}[])
                  n281 = for {
                    tunnel: w541 -> [w552] mode=indexing
                    tunnel: w539 -> [w551] mode=indexing
                    shift-right: [w550] -> _
                    shift-left: _ -> [w549]
                    n282 = call "GFG_core.vi"("Variable Name in"=w551, "Variant in"=w549, "Action"=w552) -> ("Variant Out"=w550:variant)  [unwired: 10 in, 6 out]
                  }
                }
              }
            }
            n283 = for {
              N: 1 -> [_]
              shift-right: [w554] -> _
              shift-left: _ -> [w556]
              tunnel: [w553] -> w522
              n284 = Tick Count (ms)() -> (millisecond timer value=w554:u32)
              n285 = Subtract(x=w554, y=w556) -> (x-y=w557:u32)
              n286 = Greater?(x=w557, y=u32 500) -> (0:w553:bool)
            }
            n287 = case shown="True" w522 {
              frame False {
              }
              frame True {
                n288 = call "GFG refresh all variables.vi"("Variables to refresh"=string[] ["pixel.resolution"] ("All Variable Names")) -> ()  [unwired: 11 in]
              }
            }
          }
          frame "scan.mode.main.settings" {
            n289 = Variant To Data(type=scan_mode_main_settings_tab."2D frame" ("scan mode main settings"), Variant=w564) -> (data=w562:T4)  [unwired: 1 in, 1 out]
            n290 = case shown="\"2D frame\", Default" w562 {
              tunnel: w561 -> [w578 w585 w591 w592]
              tunnel: [w578 w585 w591 w592] -> w560
              frame "2D frame", Default {
                n291 = call-poly "GFGpolyGet.vi"("Variable Name in"="y.pixels") -> ("output cluster"=w570:T2)  [unwired: 9 in, 1 out]
                n292 = Unbundle By Name(w570) -> ("DigitalRef"=w569:refnum<vi>)
                n293 = call "GFG_core.vi"("Variable Name in"="no..of.frames.for.frame.scan", "Action"=enum16{"Init", "Set", "Get"}."Get") -> ("Variable Name Out"=w573:string)  [unwired: 11 in, 6 out]
                n294 = call "line scan enable disable.vi"("Page Enabled State"=T8."Page Disabled & Grayed") -> ()  [unwired: 11 in]
                n295 = call "GFG_core.vi"("Variable Name in"="experiment type", "Variant in"=T7 "XYT" ("experiment type"), "Action"=enum16{"Init", "Set", "Get"}."Set") -> ()  [unwired: 10 in, 7 out]
                n296 = property class="DigNum"(reference=w569, "DisabledEnum"=T5."Enabled" ("Disabled")) -> ()  [unwired: 1 in, 2 out]
                n297 = call "GFG_core.vi"("Variable Name in"=" no..of.frames.to.acquire", "Variant in"=w573, "Action"=enum16{"Init", "Set", "Get"}."Set") -> ()  [unwired: 10 in, 7 out]
              }
              frame "Z Stack" {
                n298 = call "control tab sliding.vi"("close(T)/open(F)"=FALSE, "String"="advanced settings slider tab") -> ()  [unwired: 10 in]
                n299 = call "GFG_core.vi"("Variable Name in"="advanced settings inner tab", "Variant in"=advanced_settings_inner_tab_CTL."Zstack data" ("advanced settings inner tab"), "Action"=enum16{"Init", "Set", "Get"}."Set") -> ()  [unwired: 10 in, 7 out]
                n300 = call "GFG_core.vi"("Variable Name in"="experiment type", "Variant in"=T7 "XYTZ" ("experiment type"), "Action"=enum16{"Init", "Set", "Get"}."Set") -> ()  [unwired: 10 in, 7 out]
              }
              frame "2D line scan" {
                n301 = call "GFG_core.vi"("Variable Name in"="experiment type", "Variant in"=T7 "[xy]T" ("experiment type"), "Action"=enum16{"Init", "Set", "Get"}."Set") -> ()  [unwired: 10 in, 7 out]
              }
              frame "piezo" {
                n302 = Build Array("no.of.cycles.to.scan" ("Variable Name")) -> (w593:string[])
                n303 = call "GFG refresh all variables.vi"("Variables to refresh"=w593) -> ()  [unwired: 11 in]
              }
            }
          }
          frame "resonant.display.queue.to.fp.display_MD.completed", "resonant.image.queue.to.disk.and.display.queue_MD.completed", "resonant.raw.queue.to.image.queue_MD.completed", "resonant.scan.engine_MD.completed" {
            n304 = for {
              N: 1 -> [_]
              shift-right: [w620] -> _
              shift-left: _ -> [w622]
              tunnel: [w621] -> w603
              n305 = Tick Count (ms)() -> (millisecond timer value=w620:u32)
              n306 = Subtract(x=w620, y=w622) -> (x-y=w621:u32)
            }
            n307 = Greater?(x=u32 1000 ("y"), y=w603) -> (0:w600:bool)
            n308 = local read "String"() -> (w599:string)
            n309 = Select(t=w599, s=w600, f="") -> (s? t:f=w601:string)
            n310 = Concatenate Strings(w601, "\r\n", w609) -> (w608:string)
            n311 = local write "String"(w608) -> ()
            n312 = for {
              tunnel: w608 -> [w629]
              tunnel: string[] ["resonant.scan.engine_MD.completed", "resonant.raw.queue.to.image.queue_MD.completed", "resonant.image.queue.to.disk.and.display.queue_MD.completed", "resonant.display.queue.to.fp.display_MD.completed"] ("appended array") -> [w628] mode=indexing
              shift-right: [w624] -> w605
              shift-left: i16 0 -> [w623]
              n313 = Match Pattern(string=w629, regular expression=w628) -> (offset past match=w627:i32)  [unwired: 1 in, 3 out]
              n314 = Greater Or Equal To 0?(x=w627) -> (x >= 0?=w626:bool)
              n315 = Boolean To (0,1)(Boolean=w626) -> (0, 1=w625:i16)
              n316 = Add(x=w625, y=w623) -> (x+y=w624:i16)
            }
            n317 = Equal?(x=w605, y=i16 4) -> (x = y?=w595:bool)
            n318 = case shown="True" w595 {
              selector: w595 -> [_ w615]
              frame False {
              }
              frame True {
                n319 = local write "String"("") -> ()
                n320 = call "MacroRules_FGV.vi"("MacroRules_FGV_Commands"=MacroRules_FGV_Commands."Get Param and Flags", "Command Name IN"="Record") -> ("Flags"=w612:string[])  [unwired: 5 in, 4 out]
                n321 = for {
                  tunnel: w612 -> [w618] mode=indexing
                  n322 = call "GFG_core.vi"("Variable Name in"=w618, "Variant in"=TRUE, "Action"=enum16{"Init", "Set", "Get"}."Set") -> ()  [unwired: 10 in, 7 out]
                }
                "ready for flystart?" <- w615
              }
            }
          }
          frame "MAIN.Image.panels.reso." {
            n323 = Variant To Data(type=MAIN_Image_panel_reso_tab_Control_type_def."Channel 2" ("MAIN Image panels reso"), Variant=w640) -> (data=w639:T6)  [unwired: 1 in, 1 out]
            n324 = call-poly "GFGpolyGet.vi"("Variable Name in"="Histograms tab reso") -> ("output cluster"=w636:T2)  [unwired: 9 in, 1 out]
            n325 = Unbundle By Name(w636) -> ("TabControlRef"=w634:refnum<vi>)
            n326 = feedback #4() -> (w630:T11)  [unwired: 1 in]
            n327 = case shown="\"all channels\"" w639 {
              tunnel: w638 -> [w646 w652 w658 w664 w670 w672]
              tunnel: [w646 w652 w658 w664 w670 w672] -> w637
              tunnel: [Histogram_tab_reso."hist Ch 1" ("Histograms tab reso") Histogram_tab_reso."hist Ch 2" ("Histograms tab reso") Histogram_tab_reso."hist Ch 3" ("Histograms tab reso") Histogram_tab_reso."hist Ch 4" ("Histograms tab reso") Histogram_tab_reso."hist Ch 5" ("Histograms tab reso") w671] -> w631
              tunnel: w630 -> [_ _ _ _ _ w671]
              frame "Channel 1", Default {
                n328 = call-poly "GFGpolyGet.vi"("Variable Name in"="autocorrect.startdelay") -> ("output cluster"=w643:T2)  [unwired: 9 in, 1 out]
                n329 = Unbundle By Name(w643) -> ("BooleanRef"=w642:refnum<vi>)
                n330 = property class="Bool"(reference=w642, "DisabledEnum"=T5."Enabled" ("Disabled")) -> ()  [unwired: 1 in, 2 out]
              }
              frame "Channel 2" {
                n331 = call-poly "GFGpolyGet.vi"("Variable Name in"="autocorrect.startdelay") -> ("output cluster"=w649:T2)  [unwired: 9 in, 1 out]
                n332 = Unbundle By Name(w649) -> ("BooleanRef"=w648:refnum<vi>)
                n333 = property class="Bool"(reference=w648, "DisabledEnum"=T5."Enabled" ("Disabled")) -> ()  [unwired: 1 in, 2 out]
              }
              frame "Channel 3" {
                n334 = call-poly "GFGpolyGet.vi"("Variable Name in"="autocorrect.startdelay") -> ("output cluster"=w655:T2)  [unwired: 9 in, 1 out]
                n335 = Unbundle By Name(w655) -> ("BooleanRef"=w654:refnum<vi>)
                n336 = property class="Bool"(reference=w654, "DisabledEnum"=T5."Enabled" ("Disabled")) -> ()  [unwired: 1 in, 2 out]
              }
              frame "Channel 4" {
                n337 = call-poly "GFGpolyGet.vi"("Variable Name in"="autocorrect.startdelay") -> ("output cluster"=w661:T2)  [unwired: 9 in, 1 out]
                n338 = Unbundle By Name(w661) -> ("BooleanRef"=w660:refnum<vi>)
                n339 = property class="Bool"(reference=w660, "DisabledEnum"=T5."Enabled" ("Disabled")) -> ()  [unwired: 1 in, 2 out]
              }
              frame "Channel 5" {
                n340 = call-poly "GFGpolyGet.vi"("Variable Name in"="autocorrect.startdelay") -> ("output cluster"=w667:T2)  [unwired: 9 in, 1 out]
                n341 = Unbundle By Name(w667) -> ("BooleanRef"=w666:refnum<vi>)
                n342 = property class="Bool"(reference=w666, "DisabledEnum"=T5."Enabled" ("Disabled")) -> ()  [unwired: 1 in, 2 out]
              }
              frame "all channels" {
                n343 = call-poly "GFGpolyGet.vi"("Variable Name in"="autocorrect.startdelay") -> ("output cluster"=w675:T2)  [unwired: 9 in, 1 out]
                n344 = Unbundle By Name(w675) -> ("BooleanRef"=w674:refnum<vi>)
                n345 = property class="Bool"(reference=w674, "DisabledEnum"=T5."Disabled and Grayed Out" ("Disabled")) -> ()  [unwired: 1 in, 2 out]
              }
            }
            n346 = feedback-in #4(w631) -> ()
            n347 = property class="TabCtl"(reference=w634, "Value"=w631) -> ()  [unwired: 1 in, 2 out]
          }
          frame "piezo.active" {
            n348 = Variant To Data(type=TRUE, Variant=w693) -> (data=w686:bool)  [unwired: 1 in, 1 out]
            n349 = Select(t=T5."Disabled and Grayed Out" ("Disabled"), s=w686, f=T5."Enabled" ("Disabled")) -> (s? t:f=w677:T5)
            n350 = call-poly "GFGpolyGet.vi"("Variable Name in"="Laser.Power") -> ("output cluster"=w690:T2)  [unwired: 9 in, 1 out]
            n351 = call-poly "GFGpolyGet.vi"("Variable Name in"="blanking\npercentage") -> ("output cluster"=w682:T2)  [unwired: 9 in, 1 out]
            n352 = call-poly "GFGpolyGet.vi"("Variable Name in"="enable set power max") -> ("output cluster"=w679:T2)  [unwired: 9 in, 1 out]
            n353 = Unbundle By Name(w690) -> ("KnobRef"=w689:refnum<vi>)
            n354 = Unbundle By Name(w682) -> ("DigitalRef"=w683:refnum<vi>)
            n355 = Unbundle By Name(w679) -> ("BooleanRef"=w678:refnum<vi>)
            n356 = property class="Knob"(reference=w689, "DisabledEnum"=w677) -> ()  [unwired: 1 in, 2 out]
            n357 = property class="DigNum"(reference=w683, "DisabledEnum"=w677) -> ()  [unwired: 1 in, 2 out]
            n358 = property class="Bool"(reference=w678, "DisabledEnum"=w677) -> ()  [unwired: 1 in, 2 out]
          }
          frame "Objective" {
            # "obj3.name = \"16x Nikon\"\nobj3.max.field.of.view = 0.00040000000    \nobj3.voltage.for.max.field.of.view = 1.700000000000 \nobj3.max.field.of.view.resonant = 0.000400000000  \nobj3.voltage.for.max.field.of.view.resonant = 5.000000000000    \nobj3.voltage.for.min.field.of.view.resonant = 3.000000000000"
            n359 = Variant To Data(type=u16 0, Variant=w709) -> (data=w704:u16)  [unwired: 1 in, 1 out]
            n360 = Increment(x=w704) -> (x+1=w707:u16)
            n361 = Number To Decimal String(number=w707) -> (decimal integer string=w696:string)  [unwired: 1 in]
            n362 = call "GFG_core.vi"("Variable Name in"="active.objective", "Variant in"=w704, "Action"=enum16{"Init", "Set", "Get"}."Set") -> ()  [unwired: 10 in, 7 out]
            n363 = Build Array("max.field.of.view", "voltage.for.max.field.of.view", "max.field.of.view.resonant", "voltage.for.max.field.of.view.resonant", "voltage.for.min.field.of.view.resonant") -> (w697:string[])
            n364 = for {
              tunnel: w697 -> [w715] mode=indexing
              tunnel: w696 -> [w718]
              tunnel: "obj" -> [w719]
              tunnel: "." -> [w717]
              n365 = Concatenate Strings(w719, w718, w717, w715) -> (w716:string)
              n366 = Build Array(w716, w715) -> (w711:string[])
              n367 = Build Array(enum16{"Init", "Set", "Get"}."Get" ("Action"), enum16{"Init", "Set", "Get"}."Set" ("Action")) -> (w712:enum16{"Init", "Set", "Get"}[])
              n368 = for {
                tunnel: w712 -> [w723] mode=indexing
                tunnel: w711 -> [w722] mode=indexing
                shift-right: [w721] -> _
                shift-left: _ -> [w720]
                n369 = call "GFG_core.vi"("Variable Name in"=w722, "Variant in"=w720, "Action"=w723) -> ("Variant Out"=w721:variant)  [unwired: 10 in, 6 out]
              }
            }
          }
          frame "shutdown" {
          }
        }
      }
      event Mouse Down {
        n370 = event-data() -> ("CtlRef"=w727:refnum<vi>)  [unwired: 1 in]
        n371 = property class="Ctl"(reference=w727) -> ("DisabledEnum"=w728:T5)  [unwired: 1 in, 2 out]
        n372 = case shown="\"Enabled\"" w728 {
          tunnel: w733 -> [w740 w742]
          tunnel: w732 -> [w739 _]
          tunnel: [w738 w742] -> w731
          tunnel: w730 -> [w737 _]
          frame "Enabled" {
            n373 = register-events(reference=w740, refnum<user-event> refnum ("user event out"), w737, w739, w739) -> (reference out=w738:refnum<event-registration>)  [unwired: 1 in, 1 out]
            n374 = call "Timer.vi"("Timer Command"=Timer_Commands."Start", "name qualifier (empty if unwired)"="mouse down timer", "Set Time IN (s)"=0.5) -> ()  [unwired: 3 in, 6 out]
          }
          frame "Disabled", Default {
          }
        }
      }
      event Mouse Leave; Mouse Up {
        n375 = event-data() -> ("CtlRef"=w745:refnum<vi>)  [unwired: 1 in]
        n376 = property class="Ctl"(reference=w745) -> ("DisabledEnum"=w744:T5)  [unwired: 1 in, 2 out]
        n377 = case shown="\"Enabled\"" w744 {
          tunnel: w750 -> [w763 w804]
          tunnel: w745 -> [w753 _]
          tunnel: [w761 w804] -> w749
          tunnel: w743 -> [w760 _]
          tunnel: w748 -> [w759 _]
          tunnel: w747 -> [w758 _]
          frame "Enabled" {
            n378 = call "Timer.vi"("Timer Command"=Timer_Commands."Check Time", "name qualifier (empty if unwired)"="mouse down timer", "Set Time IN (s)"=0.5) -> ("Complete?"=w757:bool)  [unwired: 3 in, 5 out]
            n379 = register-events(reference=w763, w760, w759, w759, w759) -> (reference out=w762:refnum<event-registration>, error out=w751:errorcluster)  [unwired: 1 in]
            n380 = case shown="True" w757 {
              tunnel: w753 -> [_ w770]
              tunnel: w751 -> [w764 w769]
              tunnel: [w764 w768] -> w752
              frame False {
              }
              frame True {
                n381 = flat-sequence {
                  tunnel: w770 -> [w797]
                  tunnel: [w792] -> w768
                  tunnel: w769 -> [w792]
                  frame #0 {
                    n382 = property class="Ctl"(reference=w797) -> ("Label.Text"=w796:string)  [unwired: 1 in, 2 out]
                    n383 = call "wait for fp element value stable.vi"("CtlRef"=w797) -> ("Value"=w795:variant)  [unwired: 9 in, 1 out]
                    n384 = call "GFG_core.vi"("Variable Name in"=w796, "Variant in"=w795, "Source VI"="calculation.vi mouse event", "Action"=enum16{"Init", "Set", "Get", "Clear"}."Set") -> ()  [unwired: 9 in, 7 out]
                  }
                }
                n385 = Build Array("Start.Delay" ("Variable Name in"), "ZOOM" ("Variable Name in")) -> (w765:string[])
                n386 = for {
                  tunnel: w765 -> [w789] mode=indexing
                  tunnel: [w771] -> _ mode=indexing
                  n387 = call-poly "GFGpolyGet.vi"("Variable Name in"=w789) -> ("output cluster"=w774:T2)  [unwired: 9 in, 1 out]
                  n388 = Unbundle(w774) -> ("WaveformChartRef"=w778:refnum<vi>, "DigitalRef"=w779:refnum<vi>, "ArrayRef"=w780:refnum<vi>, "TabControlRef"=w781:refnum<vi>, "EnumRef"=w782:refnum<vi>, "RingRef"=w783:refnum<vi>, "BooleanRef"=w784:refnum<vi>, "KnobRef"=w785:refnum<vi>, "SlideRef"=w786:refnum<vi>, "PathRef"=w787:refnum<vi>, "StringRef"=w788:refnum<vi>, "ComboBox"=w777:refnum<vi>, "WaveformGraphRef"=w776:refnum<vi>)
                  n389 = Build Array(w778, w779, w780, w781, w782, w783, w784, w785, w786, w787, w788, w777, w776) -> (w775:refnum<vi>[])
                  n390 = for {
                    tunnel: w775 -> [w790] mode=indexing
                    tunnel: [w790] -> w772
                    stop <- w791 continue-if-true
                    n391 = Not A Number/Path/Refnum?(number/path/refnum=w790) -> (NaN/Path/Refnum?=w791:bool)
                  }
                  n392 = property class="Ctl"(reference=w772, "DisabledEnum"=T5."Disabled and Grayed Out" ("Disabled")) -> (error out=w771:errorcluster)  [unwired: 1 in, 1 out]
                }
              }
            }
            n393 = flat-sequence {
              tunnel: w762 -> [w803]
              tunnel: [w802] -> w761
              tunnel: w760 -> [w801]
              tunnel: w759 -> [w799]
              tunnel: [w800] -> _
              tunnel: w758 -> [w798]
              tunnel: w752 -> [_]
              frame #0 {
                n394 = register-events(reference=w803, w801, w798, w799, w799) -> (reference out=w802:refnum<event-registration>, error out=w800:errorcluster)  [unwired: 1 in]
              }
            }
          }
          frame "Disabled", Default {
          }
        }
      }
    }
    "Iteration" <- w84
  }
